vi "Ballistics_PBBA_alpha.vi"() -> ()   [LabVIEW 2012]
doc: "This program is currently beta software. It is designed to address the data requirements defined primarily by the DHB Ballistic Test Report.\n\nThe general operation of this program is based on the Ballistics Version 2005 application developed internally by DuPont as a research tool for the Spruance Plant Ballistics Lab in Richmond, VA.\n\nPlease note that the original trigger control logic was modified and no longer depends on a safety interlock system to enable operation of a ballistic test.\n\nDuPont makes no warranties and assumes no liabilities in connection with any use of this program."
uses:
  <vilib>/Utility/NIReport.llb/NI_report.lvclass
  <vilib>/addons/database/NI_Database_API.lvlib
  <vilib>/addons/database/Connection.llb/Conn Execute.vi
  <vilib>/addons/database/Recordset.llb/Rec Destroy - Connection.vi
  <vilib>/Utility/config.llb/NI_LVConfig.lvlib
  <vilib>/Utility/config.llb/Write Key (I32).vi
  <vilib>/addons/database/Connection.llb/DB Tools Open Connec (String).vi
  <vilib>/Analysis/NI_AALBase.lvlib
  Instance           1 29Saved   Ballistics_PBBA_alpha .vi
  <vilib>/Utility/NIReport.llb/Append Text Table to Report (wrap).vi
  <vilib>/Utility/NIReport.llb/Append Report Text (str wrap).vi
  Shot Record.ctl
panel:
  out "dbConn":string caption="Database Connection"
  in  "RESET":bool
  in  "EXIT":bool
  in  "message control":bool=TRUE
  in  "String":string="Ply Data Not Entered"
  in  "mainTabCntrl":T1(tab)=enum."MEASURE"
  in  "setupTabCntrl":T2(tab)
  in  "weight(gr)":u16(ring) caption="Weight (gr)" items=["2", "4", "16", "17", "44", "64", "124", "158", "240"]
  in  "clayAverage":sgl caption="Clay Average"
  in  "clayCalib":string="##-##-##-##-##" caption="Calibration"
  in  "clayTemp":i16=65 caption="Clay Temperature"
  in  "Room Temperature":i32
  in  "Room Humidity":i32
  in  "Sample ID":string
  in  "Test Conditions":u16(ring) items=["Dry", "Wet", "Hot 160 DEG. F", "Cold", "WEAPON LUBRICANT", "MOTOR OIL", "CONDITIONED", "ACCELERATED AGEING"]
  in  "Panel Dimensions":u16(ring) items=["15x15", "HELMET", "12x15", "16X16", "18X18", "20X16", "15x18", "24x24", "13X13", "7.5x7.5", "VEST PANEL", "12X12", "101/4x113/4", "15X16", "26X26", "NOT APPLICABLE", "8.5x11", "CHEST PLATE"]
  in  "Submitter":u16(ring) items=["other"]
  in  "Test Comments":string
  in  "Panel Backing":u16(ring)=1 items=["miscellaneous", "Clay (ROMA Plastilina # 1)", "Aluminum, 24 ga. (.020,.2024-T3) Witness Plate", "None"]
  in  "Threat 2":u16(ring) caption="Threat" items=["16-grain,  saboted RCC,.308cal.SAAMI test bbl.,DC", "17-grain,sabot.Type 1,FSP,.308cal.SAAMI test bbl.,DC", "17-grain,sabot.Type 2,FSP,.308cal.SAAMI test bbl.,DC", "2-grain, saboted RCC FSP,.223cal.SAAMI test bbl.,DC", "4-grain, saboted RCC FSP ,.223cal.SAAMI test bbl.,DC", "44-grain,sabot.      FSP,.458cal.SAAMI test bbl.,DC", "64-grain,sabot.  RCC,.458cal.SAAMI test bbl.,DC"]
  in  "recorder":u16(ring) caption="Recorder" items=["Mike Slate", "Dan Kraus", "Pat Fitzgerald", "Other"]
  in  "shooter":u16(ring) caption="Shooter" items=["Mike Slate", "Pat Fitzgerald", "Other"]
  in  "rangeNum":u16(ring) caption="Range #" items=["1", "2", "Other"]
  in  "barrelLen":u16(ring) caption="Barrel Length" items=["24", "10", "Other"]
  in  "projectile":u16(ring) caption="Projectile" items=["RCC", ".357mag JSP", ".44mag SJHP", "9mm FMJ", "22cal FSP", "7.62 FMJ"]
  in  "weapon":u16(ring) caption="Weapon" items=["Universal Receiver", "Other"]
  in  "minV50":i32=1500 caption="Minimum V50"
  in  "covering":u16(ring) caption="Ballistic Cover" items=["Other", "RipStop"]
  out "totalBAW":sgl caption="Total BAW" format="%.2f"
  in  "totalSampleWt":sgl caption="Total Weight" format="%.2f"
  in  "modelNum":string caption="Model #"
  in  "serialNum":string caption="Serial #"
  in  "workType":u16(ring) caption="Type of Work" items=["R&D", "QC", "Other"]
  in  "projNum":string caption="Project #"
  in  "projName":string caption="Project Name"
  in  "standard":u16(ring)=1 caption="Standard" items=["NIJ 0101.04", "MIL-STD-662F", "Other"]
  in  "Powder Type":u16(ring) items=["WINCHESTER-231", "Alliant Herc. Bullseye", "Power Pistol", "ACCURATE, NO.9", "ACCURATE, NO. 2", "IMR-4756", "OTHER", "WINCHESTER-296", "Alliant 2400", "IMR-4198", "IMR-4895", "Hi-Skor 700x", "Hi-Skor 800x", "International Clay's", "Winchester Ball", "Hercules"]
  in  "ballistician":u16(ring) caption="Ballistician" items=["n.a."]
  in  "Method":u16(ring) items=["V50", "N.I.J.", "Quasi N.I.J.", "VsVr", "CUSUM", "V(0)", "V(0) @ 1450", "V(0) @ 1500", "V(0) @ 1550"]
  out "fab6_totalWt":sgl caption="Fab6 Wt" min=0 max=99 step=5 format="%.2f"
  out "fab5_totalWt":sgl caption="Fab5 Wt" min=0 max=99 step=5 format="%.2f"
  out "fab4_totalWt":sgl caption="Fab4 Wt" min=0 max=99 step=5 format="%.2f"
  out "fab3_totalWt":sgl caption="Fab3 Wt" min=0 max=99 step=5 format="%.2f"
  out "fab2_totalWt":sgl caption="Fab2 Wt" min=0 max=99 step=5 format="%.2f"
  out "fab1_totalWt":sgl caption="Fab1 Wt" min=0 max=99 step=5 format="%.2f"
  in  "Layers":T3(array[cluster])=[{"Ply Description"=0, "Layer Comments"="", "Number of Plies"=20, "Fabric.vendor"=1, "Fabric.styleNum"=1, "Fabric.fiber"=1, "Fabric.denier"=1, "Fabric.pickWeave"=0, "Fabric.finish"=0, "LotNum"="n/a", "RollNum"="n/a", "ozPerYd2"=20.0, "Fabric.stitch"=0}] {"Fabric.stitch" items=["Corners", "Other", "n/a"]; "ozPerYd2" min=0 max=99 step=5; "Fabric.finish" items=["Greige", "ML", "WRT", "Other"]; "Fabric.pickWeave" items=["18x18 / Plain", "20x20 / Plain", "24x24 / Stn,Pln,Sn", "Other"]; "Fabric.denier" items=["600", "800", "840", "1000", "Other"]; "Fabric.fiber" items=["Kevlar", "Twaron", "Other"]; "Fabric.styleNum" items=["8606", "A087", "8542B", "Other"]; "Fabric.vendor" items=["TTI", "Barrday", "TexTech", "Other"]; "Number of Plies" min=0 max=99 step=5; "Ply Description" items=["ANY STYLE", "none"]}
  in  "Fabric Description":string
  out "Total Number of Layers":i32=1 caption="Total Number\nof Layers" min=0 max=100 step=5
  in  "Panel Technician":u16(ring) items=["Not Known", "none", "POINT BLANK"]
  in  "Weight of Panel":dbl format="%.4f"
  in  "Areal density text":string
  in  "Areal Density":dbl format="%.2f"
  in  "Thickness":dbl format="%.2f"
  in  "Manufacturer":u16(ring) caption="Mfr" items=["Point Blank-Marine Interceptor", "Other"]
  in  "Type":u16(ring) items=["none"]
  in  "Panel Type":u16(ring) items=["FABRIC ARMOR", "COMPOSITE ARMOR", "LG.RIGHT FRONT VEST PANEL", "HELMET", "N.A."]
  in  "Panel Stitch":u16(ring) items=["TEST PANEL/NORMAL STITCH", "TEST PANEL/CUSTOM STITCH", "VEST PANEL/CUSTOM STITCH", "HARD PANEL", "CAR ARMOR LAMINATE PANEL", "N.A."]
  in  "Next Shot":bool
  in  "Delete Button":bool
  in  "SHOTS":T4[](array[typedef]) {"UncorrectedAvgVel_PB" format="%.1f"; "strikeVel_PB" format="%.1f"; "velLoss_PB" format="%.1f"; "avgVel_PB" format="%.1f"; "Redundant_Velocity" format="%.1f"; "Energy Loss (J)" format="%.3e"; "Projectile Mass" min=0 step=1 format="%.4f"; "Corrected residual" format="%.2f"; "Uncorrected Residual" format="%.2f"; "Corrected Impact" format="%.2f"; "Uncorrected Impact" format="%.2f"; "Shot Angle" max=90 step=1; "SHOT STATUS" items=["Partial", "Complete"]; "IMPACT VELOCITY" min=0 max=10000 step=0.1 format="%.1f"; "Barrel Temperature" format="%.1f"; "Powder Loading" format="%.4f"; "RESIDUAL  VELOCITY" min=0 max=10000 step=0.1 format="%.1f"}
  in  "reread":bool
  out "Shot":i32
  out "Panel":i32
  out "rangeOfResults":i32 caption="Range of Results" min=0 max=10000 step=1
  out "lowComplete":i32 caption="LOW Complete" min=0 max=10000 step=1
  out "highPartial":i32 caption="HIGH Partial" min=0 max=10000 step=1
  out "Avg/speed":sgl caption="Average" min=0 max=10000 step=0.1 format="%.1f"
  in  "Current/avg/speed":sgl caption="REDUNDANT VELOCITY" min=0 max=1000000 step=0.1 format="%.1f"
  out "Redundant/speed":sgl caption="Chronograph 2" min=0 max=10000 step=0.1 format="%.1f"
  in  "backfacedia":sgl
  in  "backdepth":sgl
  out "% Difference":sgl=0.991641 format="%.1f"
  out "zmr 2":sgl caption="Z.M.R." format="%.1f"
  out "Pairs":i16 min=0 max=100 step=1
  out "computed_V50":sgl caption="Value" format="%.1f"
  in  "MaxDeviation":sgl=125.0 caption="Maximum\nDeviation" min=0 max=200 step=25 format="%.1f"
  in  "B.F.S (mm)":u16 caption="B.F.S"
  in  "N.I.J":u16(ring) items=["Not Tested", "PASS", "FAIL"]
  in  "Projectile Mass":sgl=7.12788 caption="Projectile Mass\n(grams)" min=0 step=1 format="%.4f"
  in  "Shot Angle":u16 max=90 step=1
  in  "Powder Loading":sgl min=0 max=100 step=0.1 format="%.3f"
  in  "Shot Decription":string
  in  "Barrel Temp":sgl format="%.1f"
  out "Residual factor":sgl=1.0 caption="Residual" min=0 max=1 format="%.5f"
  out "Impact factor":sgl=1.0 caption="Impact" min=0 max=1 format="%.5f"
  out "DC_ factor":sgl=1.0 caption="Midpoint of\nChrono 1 and 2" format="%.4f"
  in  "Drag Corrected":bool=TRUE
  in  "Current/redundant/speed":sgl caption="REDUNDANT VELOCITY" min=0 max=1000000 step=0.1 format="%.1f"
  out "currentDateTime":string
  in  "Current/residual/speed":sgl min=0 max=10000 step=0.1 format="%.1f"
  in  "Current/sthotstatus":u16(ring) items=["Partial", "Complete"]
  in  "Current/impact/speed":sgl min=0 max=10000 step=0.1 format="%.1f"
  out "BACKFACE DEPTH":sgl caption="Backface\nDepth" min=0 max=200 step=5
  out "BACKFACE DIAMETER":sgl caption="Backface\nDiameter" min=0 max=100 step=5
  in  "Reject shot":bool
  in  "Accept Data":bool
  out "SUBMIT DATE/TIME":string
  out "residual/speed":sgl caption="Residual" min=0 max=10000 step=0.1 format="%.1f"
  out "SHOT STATUS":u16(ring) caption="Penetration" items=["Partial", "Complete"]
  out "Impact/speed":sgl caption="Chronograph 1" min=0 max=10000 step=0.1 format="%.1f"
  in  "Table of Shots":string[][](table) caption="Shot Table"
  in  "RANGE RESET":bool
  in  "Save":bool
  out "Data retrieval":string="\nWORKING"
  out "ActualNumRecs":i32=1001 caption="Actual Number of \nRecords Returned"
  in  "latest Date":string="1/1/2100"
  in  "DATE 3":string="1/1/2100"
  in  "DATE 2":string="1/1/1900"
  in  "velocity-loading":bool
  in  "Panel Search":bool
  in  "Earliest Date":string="1/1/1900"
  in  "maxRecs":u16=1001 min=1 max=10000 step=100
  out "v50 data 2":string[][](table)
  out "In Control":bool=TRUE caption="Control Status"
  in  "queryThreat":u16(ring) caption="Threat" items=["115-GRAIN,9mm LUGER,REFERENCE ROUND,10\" .38 cal TEST BBL.", "158-grain,WIN. 357 MAG, JHP REFERENCE ROUND, 10\" SAMMI TEST BBL.", "180-grain,WIN. 308 POWER-POINT REFERENCE ROUND, 308 TEST BBL.", "240-grain,REM. .44 mag, JSP REFERENCE ROUND, 8\" SAMMI TEST BBL."]
  in  "Powder":string="bul"
  out "St. Deviation":dbl=31.606020957071 format="%.1f"
  out "Latest Velocity":dbl=1314.9 format="%.1f"
  out "Average Velocity":dbl=1297.749514563107 format="%.1f"
  out "Previous V50 Data":cluster{dbl, dbl, dbl[][]}(graph)={0.0, 1.0, []}
  in  "Threat":string
  out "Velocity versus Loading":cluster{dbl[], dbl[]}(graph)
  out "v50 data":string[][](table)
  in  "Residual  Timer":i16=2 min=0 max=3 step=1
  in  "Redundant Timer":i16=1 min=0 max=3 step=1
  in  "Impact Timer":i16 min=0 max=3 step=1
  in  "DAQ Card":i16=1
  out "Device S/N":string caption="Timing Device S/N"
  in  "switch":bool
  in  "Stop Program":bool
  in  "old drag":bool
  out "Partial":sgl[](array[numeric]) format="%.2f"
  out "factor array":sgl[](array[numeric]) format="%.4f"
  out "Complete":sgl[](array[numeric]) format="%.2f"
  in  "Contact Shot Report":bool
  in  "Old_Shots":T4[](array[typedef]) {"UncorrectedAvgVel_PB" format="%.1f"; "strikeVel_PB" format="%.1f"; "velLoss_PB" format="%.1f"; "avgVel_PB" format="%.1f"; "Redundant_Velocity" format="%.1f"; "Energy Loss (J)" format="%.3e"; "Projectile Mass" min=0 step=1 format="%.4f"; "Corrected residual" format="%.2f"; "Uncorrected Residual" format="%.2f"; "Corrected Impact" format="%.2f"; "Uncorrected Impact" format="%.2f"; "Shot Angle" max=90 step=1; "SHOT STATUS" items=["Partial", "Complete"]; "IMPACT VELOCITY" min=0 max=10000 step=0.1 format="%.1f"; "Barrel Temperature" format="%.1f"; "Powder Loading" format="%.4f"; "RESIDUAL  VELOCITY" min=0 max=10000 step=0.1 format="%.1f"}
  in  "old threat":u16
  out "Z.M.R.":sgl min=0 step=0.1 format="%.1f"
  in  "Residual/Target Dist":sgl=7.083333 format="%.2f"
  out "Residual/Separation":sgl=4.0 format="%.2f"
  in  "Impac/Target Dist":sgl=7.083333 format="%.2f"
  out "Barrel to Screen Distance":sgl=7.8333 format="%.2f"
  out "Impact/Separation":sgl=4.0 format="%.2f"
  out "plytypes":u16=1
  out "Corrected Impact":sgl=44.292404 format="%.2f"
  out "Corrected Residual":sgl format="%.2f"
  out "correction coefficient":sgl format="%.8f"
  out "Red/ID":u32=84017153 format="%.0x"
  out "residual/ID":u32=83951617 format="%.0x"
  out "impact/ID":u32=83886081 format="%.0x"
  in  "Version":dbl format="%.2f"
  in  "percent warning":sgl=1.0 format="%.2f"
  out "number of partials":i32=2
  out "number of completes":i32=3
  out "conversion factor":sgl=0.3048037 format="%.5f"
  in  "mid_to_targ_dist":sgl caption="Midpoint To Target Distance"
  out "Corrected Redundant":sgl=44.292404 format="%.2f"
  out "Corrected Average":sgl=44.292404 format="%.2f"
  out "Shot Graph":cluster{i32[], sgl[]}[](graph)
  in  "Data Source":u16(ring)=2 items=["Simulated", "Radar", "Screens"]
  out "Distance Units":string
  out "Weight Units":string
  in  "Report_PB":bool caption="Report"
  in  "Add Disclaimer":bool
  in  "Report":bool
  in  "Report Path":path=path "c:/ballistics"
  # "The bottom section of this pane contains new fields\nspecified by the PBBA Test reports.\n\nSome of the fields from the DuPont grouping (as marked \nin the top section) are also needed to complete a report."
  # "GENERAL"
  # "SAMPLE"
  # "THREAT"
  # "RANGE"
  # "lbs."
  # "° F"
  # "lbs."
  # "mm"
  # "mm"
  # "Strike Face -------------------------------------------------------- Model Construction --------------------------------------------------------> Body Side"
  # "[----- Fabric #1 -------------- Fabric #2 -------------- Fabric #3 -------------- Fabric #4 -------------- Fabric #5 -------------- Fabric #6 -----]"
  # "Ply Description"
  # "Layer Comments"
  # "# of Plies"
  # "Vendor"
  # "Style #"
  # "Fiber"
  # "Denier"
  # "Pick / Weave"
  # "Finish"
  # "Lot#"
  # "Roll#"
  # "oz/yd²"
  # "Stitch"
  # "Total Weight"
  # "Edit any non-date field by placing cursor in field. \n\nProperties not listed are controlled by the current shot, test description or Fabric information.  \nIf the entry is changed for the current shot, then all previous shots are changed"
  # "Current Shot Data"
  # "(mm)"
  # "V50"
  # "NOTE: Number of  plies must be entered in FABRIC INFORMATION to enable saving"
  # "Point Blank Body Armor Ballistics Test Station"
  # "Last Assigned\nRecord Numbers"
  # "Correction Factors"
  # "CUSUM HISTORY"
  # "SHOT DATA"
  # "Max Records Returned\n (up to 10,000)"
  # "Date Range"
  # "(Form: 1/25/2000)"
  # "Date Range"
  # "Begin date"
  # "End Date"
  # "(Form: 1/25/2000)"
  # "End Date"
  # "Begin Date"
  # "yes"
  # "No"
  # "PBBA"
  # "Point Blank Body Armor\nBallistics Test Station\n\nVersion 1.00 ALPHA\n\nOctober 2006"
  # "To arrange for technical support, contact\n\nPat Fitzgerald or Mark Hartsky\n\nDuPont Company"
  # "This program is currently beta software. It is designed to address the data requirements defined primarily by the DHB Ballistic Test Report.\n\nThe general operation of this program is based on the Ballistics Version 2005 application developed internally by DuPont as a research tool for the Spruance Plant Ballistics Lab in Richmond, VA.\n\nPlease note that the original trigger control logic was modified and no longer depends on a safety interlock system to enable operation of a ballistic test.\n\nDuPont makes no warranties and assumes no liabilities in connection with any use of this program."
  # "Yes"
  # "No"
  # "DuPont"
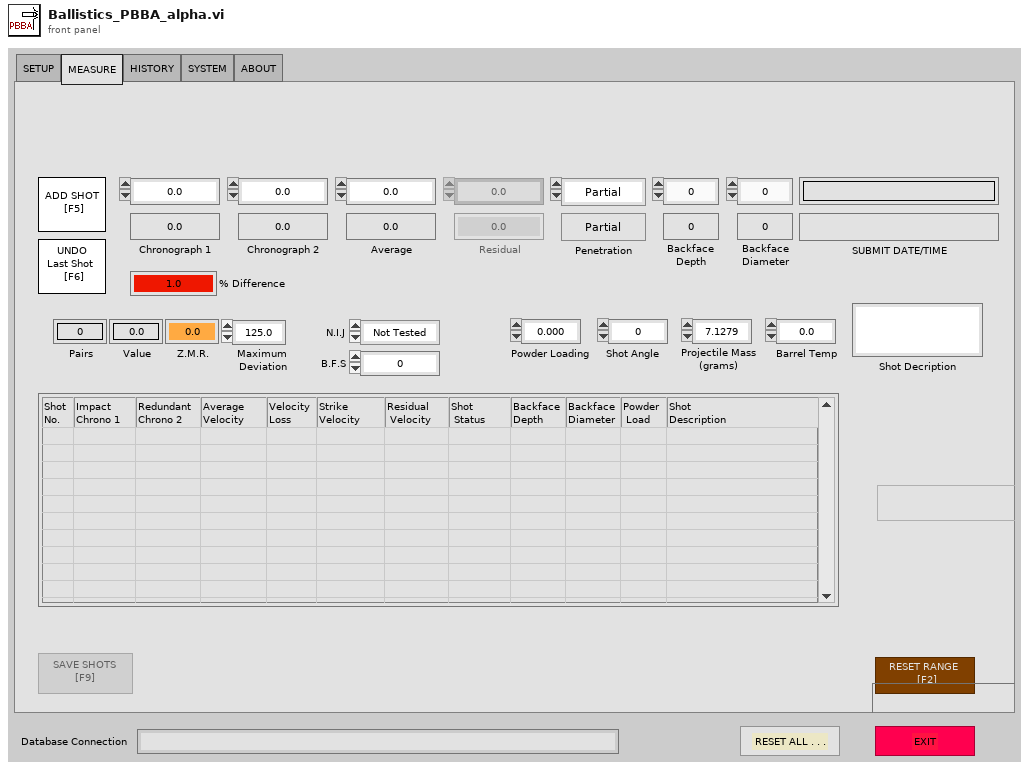
[diagram p1: front panel]
types:
  T1 = enum32{"SETUP", "MEASURE", "HISTORY", "SYSTEM", "ABOUT"}
  T2 = enum32{"Test Description", "Fabric Information", "Edit Previous Shots"}
  T3 = cluster{"Ply Description":u16, "Layer Comments":string, "Number of Plies":i32, "Fabric.vendor":u16, "Fabric.styleNum":u16, "Fabric.fiber":u16, "Fabric.denier":u16, "Fabric.pickWeave":u16, "Fabric.finish":u16, "LotNum":string, "RollNum":string, "ozPerYd2":sgl, "Fabric.stitch":u16}[]
  T4 = typedef "Shot Record.ctl" = cluster{"avgVel_PB":sgl, "IMPACT VELOCITY":sgl, "RESIDUAL  VELOCITY ":sgl, "Shot Description":string, "Powder Loading ":sgl, "Barrel Temperature":sgl, "TIME / DATE":string, "shot order":i32, "SHOT STATUS":u16, "Shot Angle":u16, "Uncorrected Impact":sgl, "Corrected Impact":sgl, "Uncorrected Residual":sgl, "Corrected residual":sgl, "Projectile Mass":sgl, "usedv50":bool, "Energy Loss (J)":sgl, "BackFace\nDepth":sgl, "BackFace\nDiameter":sgl, "Redundant_Velocity":sgl, "velLoss_PB":sgl, "strikeVel_PB":sgl, "UncorrectedRed_PB":sgl, "CorrectedRed_PB":sgl, "UncorrectedAvgVel_PB":sgl}
  T5 = cluster{"impactCntrID":u32, "redundantCntrID":u32, "residualCntrID":u32}
  T6 = cluster{"Charset (-1)":i16, "Weight (-1)":i16, "Name":string, "Size":string}
  T7 = cluster{"Italic":enum16{"Italic Unchanged", "Italic On", "Italic Off"}, "Strike Through":enum16{"Strike Through Unchanged", "Strike Through On", "Strike Through Off"}, "Underline":enum16{"Underline Unchanged", "Underline On", "Underline Off"}, "Bold":enum16{"Bold Unchanged", "Bold On", "Bold Off"}}
  T8 = enum16{"Standard Report", "HTML", "Word", "Excel"}
  T9 = typedef "NI_Database_API.lvlib/Conn ObjectReference.ctl" = refnum<k1>
  T10 = typedef "NI_Database_API.lvlib/Rec ObjectReference.ctl" = refnum<k1>
  T11 = typedef "NI_LVConfig.lvlib/Config Data RefNum.ctl" = refnum<k1>
  T12 = cluster{"task ID out":u32, "task ID out":u32, "task ID out":u32}
  T13 = cluster{"Sample ID":string, "element":string, "element":string, "serialNum":string, "modelNum":string, string, string, string, "element":string, string}
  T14 = cluster{string, string, string, "clayCalib":string, string}
  T15 = cluster{"element":string, "element":string, "element":string, "element":string, "element":string, string, "element":string, "element":string, "element":string}
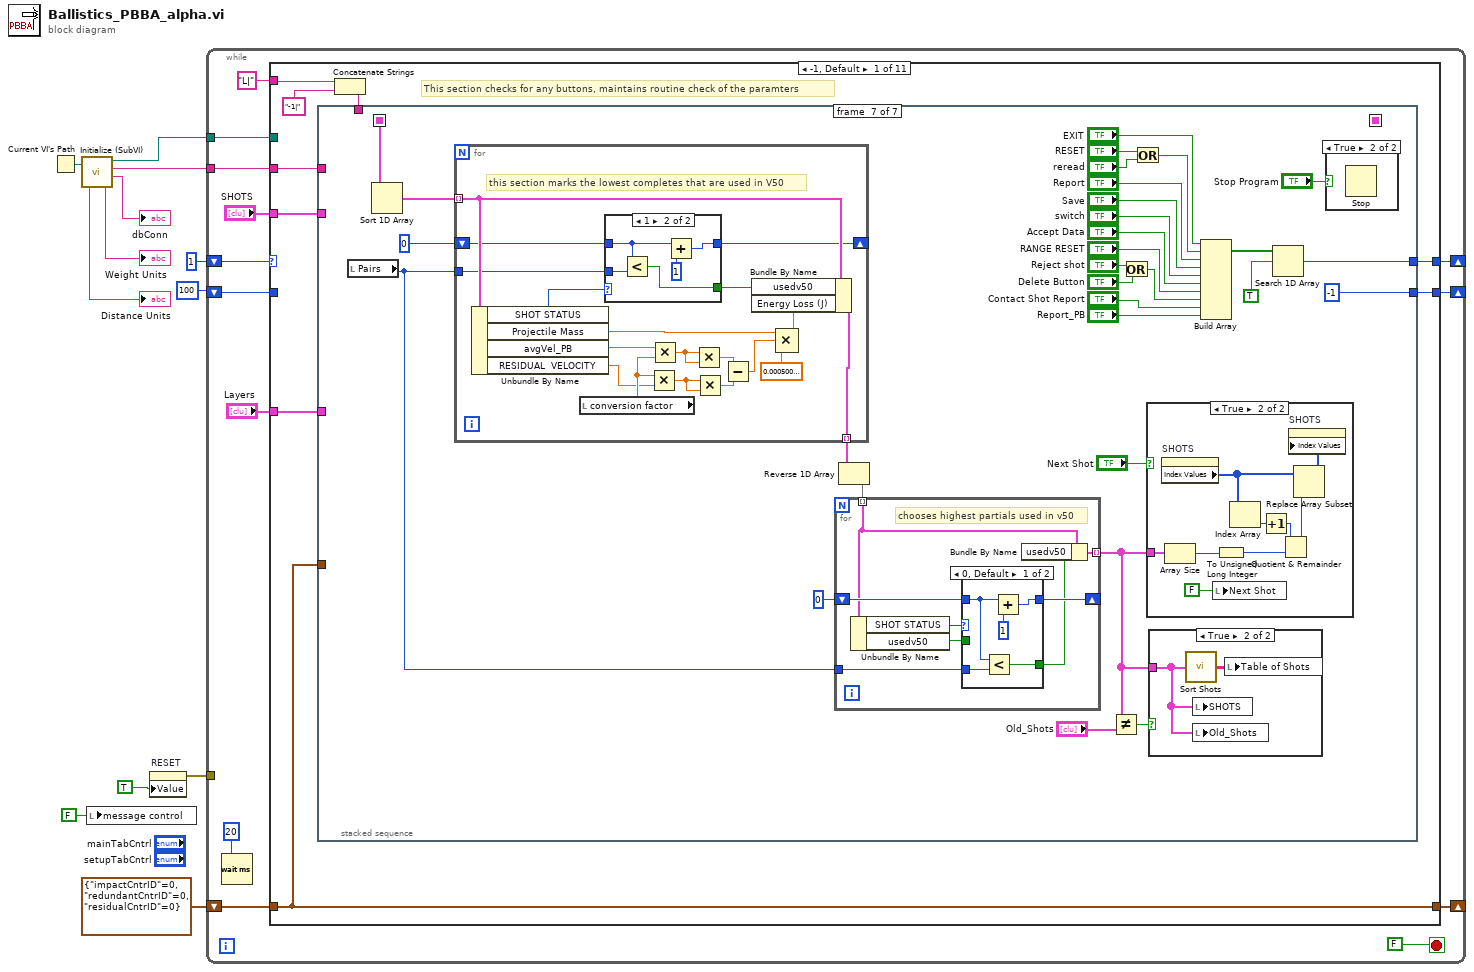
[diagram p0: block diagram]
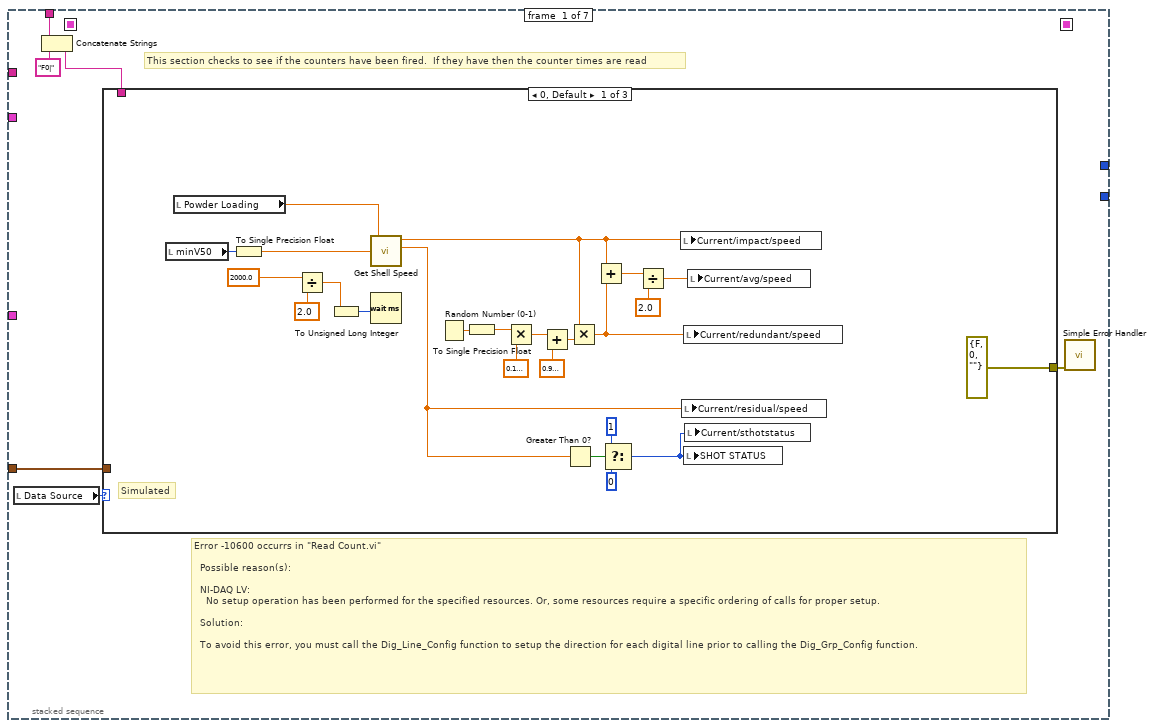
[diagram p2: hidden frame]
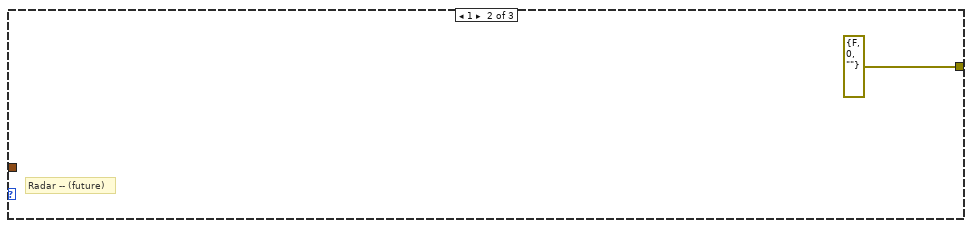
[diagram p3: hidden frame]
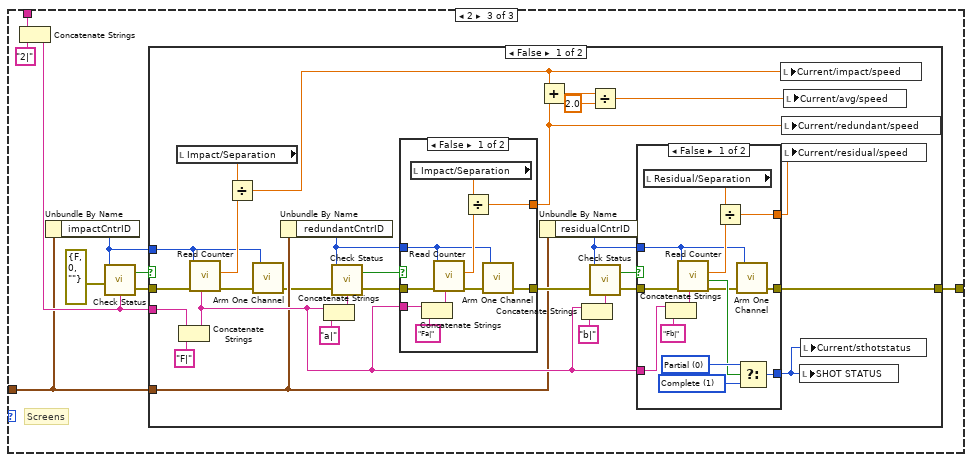
[diagram p4: hidden frame]
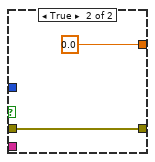
[diagram p5: hidden frame]
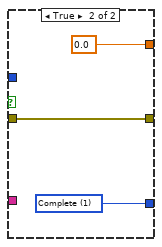
[diagram p6: hidden frame]
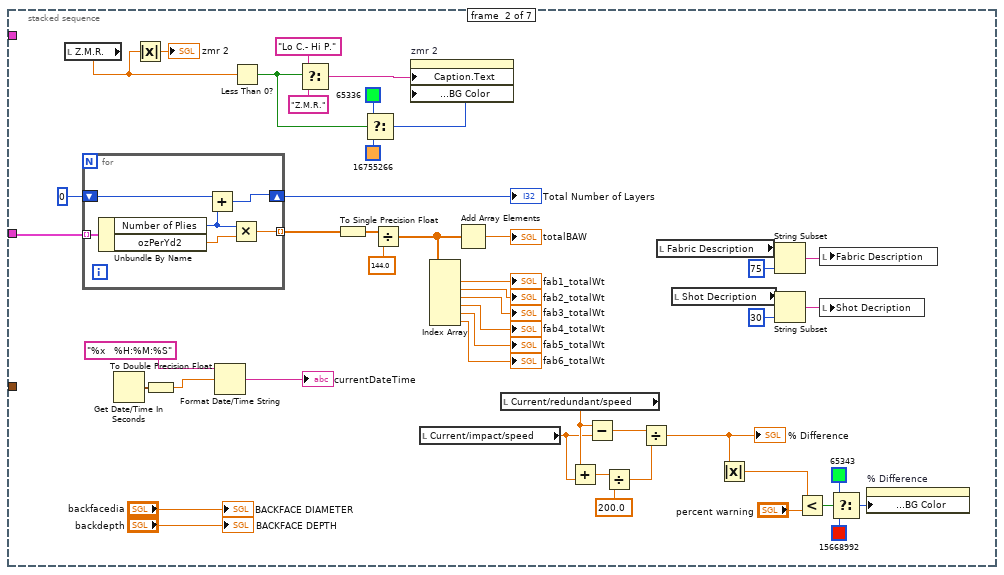
[diagram p8: hidden frame]
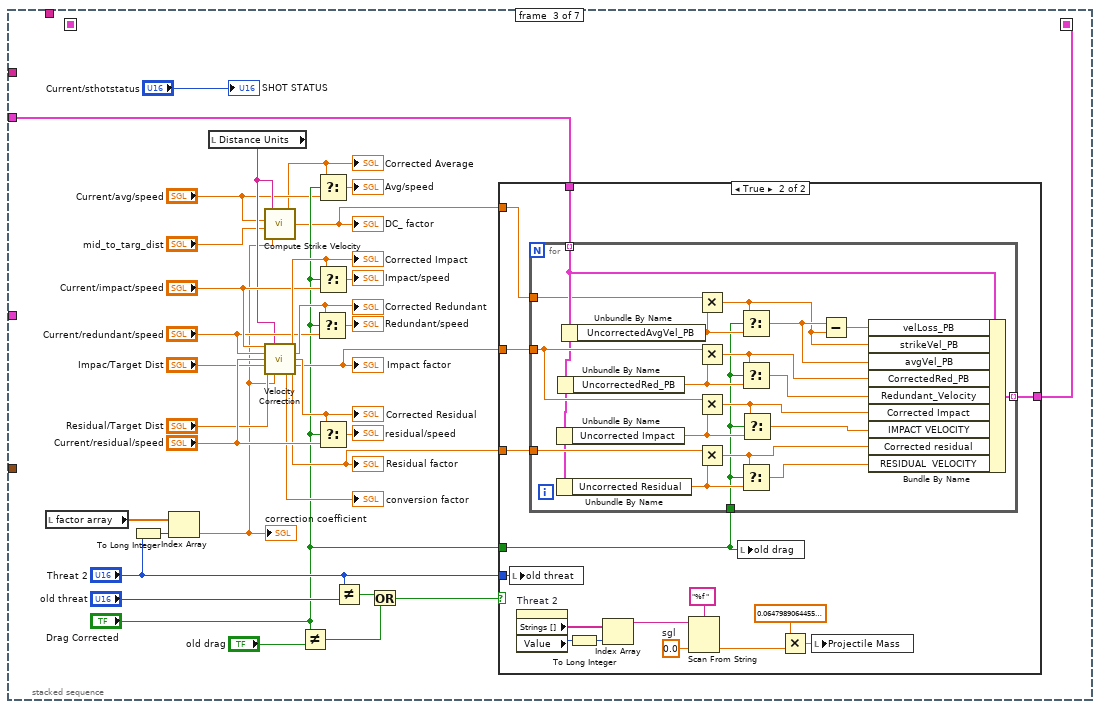
[diagram p9: hidden frame]
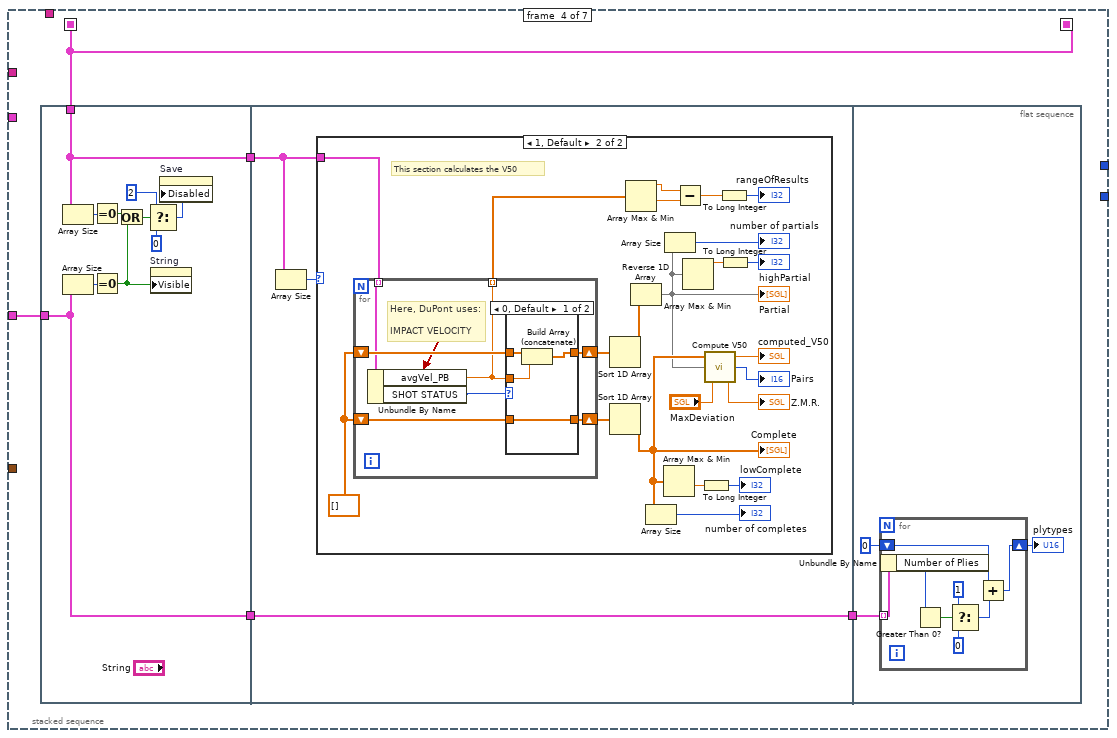
[diagram p11: hidden frame]
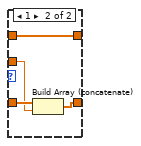
[diagram p13: hidden frame]
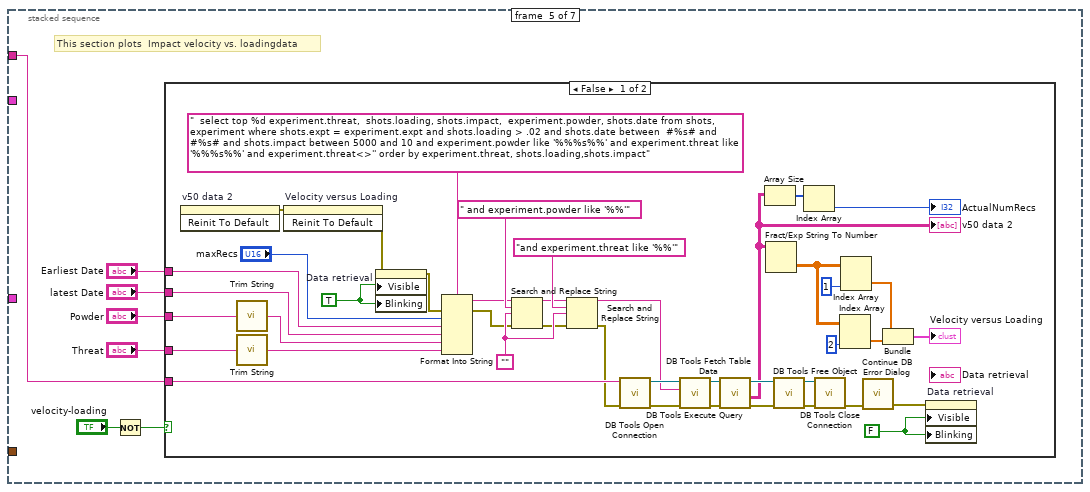
[diagram p14: hidden frame]
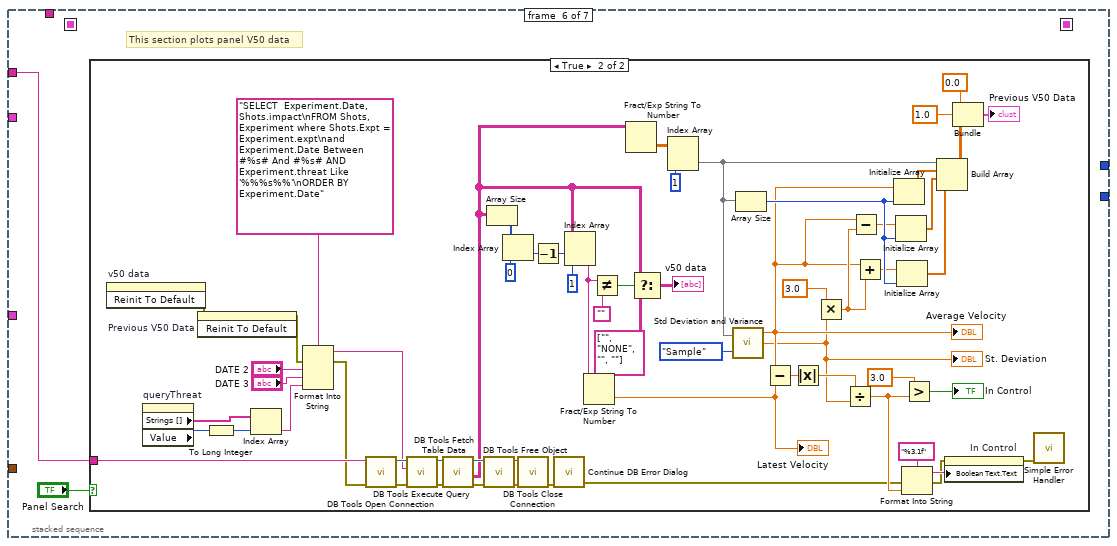
[diagram p16: hidden frame]
diagram:
  n1 = Current VI's Path() -> (path=w1:path)
  n2 = call "Initialize (SubVI).vi"("appended path IN"=w1) -> ("Distance Units"=→"Distance Units":string, "appended path OUT"=w6:path, "connectString"=w9:string, "Database Connection"=→"dbConn":string, "Weight Units"=→"Weight Units":string)
  n3 = local write "message control"(FALSE) -> ()
  n4 = property on="RESET" class="Bool (strict)"("Value"=TRUE ("RESET")) -> (error out=w7:errorcluster)  [unwired: 2 in, 1 out]
  n5 = while {
    shift-left: 100 -> [w21]
    shift-right: [w22] -> _
    shift-left: 1 ("index of element") -> [w25]
    shift-right: [w23] -> _
    tunnel: w6 -> [w18]
    tunnel: w9 -> [w17]
    tunnel: w7 -> [_]
    shift-right: [w15] -> _
    shift-left: T5 {"impactCntrID"=0, "redundantCntrID"=0, "residualCntrID"=0} -> [w14]
    stop <- FALSE stop-if-true
    n6 = Wait (ms)(milliseconds to wait=u32 20 ("millisecond timer value")) -> ()  [unwired: 1 out]
    n7 = case shown="-1, Default" w25 {
      tunnel: [w32 w517 w522 w751 w774 w1032 w1074 w1082 w1126 w1244 w1289] -> w23
      tunnel: [w33 w517 w522 w751 w773 w1032 w1074 w1082 w1126 w1244 w1289] -> w22
      tunnel: w21 -> [_ _ w525 _ _ _ _ _ _ _ _]
      tunnel: "SHOTS" -> [w34 _ _ _ w772 w1022 w1061 _ w1124 _ w1281]
      tunnel: w18 -> [_ _ w524 _ w766 _ _ _ _ _ _]
      tunnel: w17 -> [w31 _ w523 _ w770 _ _ _ _ _ _]
      tunnel: "L|" -> [w30 _ _ _ _ _ _ w1078 _ _ _]
      tunnel: [w27 w516 w521 w629 w769 w1020 w1048 w1077 w1121 w1175 w1288] -> w15
      tunnel: w14 -> [w27 w516 w521 w629 w769 w1020 w1048 w1076 w1121 w1175 w1288]
      tunnel: "Layers" -> [w26 _ _ _ w768 _ _ _ _ _ w1282]
      frame -1, Default {
        # "This section checks for any buttons, maintains routine check of the paramters"
        n8 = Concatenate Strings(w30, "-1|") -> (w28:string)
        n9 = stacked-sequence {
          seq-local: [_ _ _ w261 _ _ _] -> [_ _ _ _ _ _ w446]
          seq-local: [_ _ w211 _ _ _ _] -> [_ _ _ w261 _ _ _]
          tunnel: w34 -> [_ _ w198 _ _ _ _]
          tunnel: [_ _ _ _ _ _ w450] -> w32
          tunnel: [_ _ _ _ _ _ -1] -> w33
          tunnel: w31 -> [_ _ _ _ w323 w373 _]
          tunnel: w28 -> [w38 _ _ _ _ _ _]
          tunnel: w27 -> [w35 _ _ _ _ _ _]
          tunnel: w26 -> [_ w134 _ w259 _ _ _]
          frame #0 {
            # "Error -10600 occurrs in \"Read Count.vi\"\n\n  Possible reason(s):\n\n  NI-DAQ LV:\n    No setup operation has been performed for the specified resources. Or, some resources require a specific ordering of calls for proper setup.  \n\n  Solution: \n\n  To avoid this error, you must call the Dig_Line_Config function to setup the direction for each digital line prior to calling the Dig_Grp_Config function."
            # "This section checks to see if the counters have been fired.  If they have then the counter times are read"
            n10 = local read "Data Source"() -> (w40:u16)
            n11 = Concatenate Strings(w38, "F0|") -> (w36:string)
            n12 = case shown="0, Default" w40 {
              tunnel: [errorcluster {"status"=FALSE, "code"=0, "source"=""} ("error out") errorcluster {"status"=FALSE, "code"=0, "source"=""} ("error out") w74] -> w39
              tunnel: w36 -> [_ _ w70]
              tunnel: w35 -> [_ _ w66]
              frame 0, Default {
                # "Simulated"
                n13 = local read "minV50"() -> (w43:i32)
                n14 = local read "Powder Loading"() -> (w63:sgl)
                n15 = To Single Precision Float(number=w43) -> (single precision float=w42:sgl)
                n16 = Divide(x=sgl 2000.0, y=sgl 2.0 ("v50")) -> (x/y=w64:sgl)
                n17 = To Unsigned Long Integer(number=w64) -> (unsigned 32bit integer=w50:u32)
                n18 = call "Get Shell Speed.vi"("loading"=w63, "v50"=w42) -> ("impact"=w48:sgl, "residual"=w57:sgl)  [unwired: 2 in, 1 out]
                n19 = Wait (ms)(milliseconds to wait=w50) -> ()  [unwired: 1 out]
                n20 = Random Number (0-1)() -> (number: 0 to 1=w55:dbl)
                n21 = To Single Precision Float(number=w55) -> (single precision float=w49:sgl)
                n22 = Multiply(x=w49, y=sgl 0.1) -> (x*y=w54:sgl)
                n23 = Add(x=w54, y=sgl 0.95) -> (x+y=w52:sgl)
                n24 = Greater Than 0?(x=w57) -> (x > 0?=w60:bool)
                n25 = Multiply(x=w48, y=w52) -> (x*y=w47:sgl)
                n26 = Add(x=w48, y=w47) -> (x+y=w45:sgl)
                n27 = Select(t=u16 1, s=w60, f=u16 0) -> (s? t:f=w58:u16)
                n28 = Divide(x=w45, y=sgl 2.0 ("v50")) -> (x/y=w44:sgl)
                n29 = local write "Current/impact/speed"(w48) -> ()
                n30 = local write "Current/residual/speed"(w57) -> ()
                n31 = local write "Current/redundant/speed"(w47) -> ()
                n32 = local write "SHOT STATUS"(w58) -> ()
                n33 = local write "Current/sthotstatus"(w58) -> ()
                n34 = local write "Current/avg/speed"(w44) -> ()
              }
              frame 1 {
                # "Radar -- (future)"
              }
              frame 2 {
                # "Screens"
                n35 = Concatenate Strings(w70, "2|") -> (w69:string)
                n36 = Unbundle By Name(w66) -> ("impactCntrID"=w67:u32)
                n37 = call "Check Status.vi"("error in (no error)"=errorcluster {"status"=FALSE, "code"=0, "source"=""}, "TL Calling Location"=w69, "Task ID"=w67) -> ("error out"=w72:errorcluster, "Armed?"=w68:bool)  [unwired: 1 in]
                n38 = case shown="False" w68 {
                  tunnel: w72 -> [w97 w133]
                  tunnel: [w98 w133] -> w74
                  tunnel: w67 -> [w80 _]
                  tunnel: w69 -> [w93 _]
                  tunnel: w66 -> [w83 _]
                  frame False {
                    n39 = local read "Impact/Separation"() -> (w101:sgl)
                    n40 = Concatenate Strings(w93, "F|") -> (w88:string)
                    n41 = call "Read Counter.vi"("TL Calling Location"=w88, "error In"=w97, "TASK ID"=w80) -> ("error out"=w82:errorcluster, "time (secs)"=w103:sgl)  [unwired: 3 in, 2 out]
                    n42 = Divide(x=w101, y=w103) -> (x/y=w76:sgl)
                    n43 = call "Arm One Channel.vi"("error IN"=w82, "task ID IN"=w80) -> ("error out"=w81:errorcluster)  [unwired: 2 in, 1 out]
                    n44 = Unbundle By Name(w83) -> ("redundantCntrID"=w85:u32)
                    n45 = Concatenate Strings(w88, "a|") -> (w91:string)
                    n46 = call "Check Status.vi"("error in (no error)"=w81, "TL Calling Location"=w91, "Task ID"=w85) -> ("error out"=w96:errorcluster, "Armed?"=w87:bool)  [unwired: 1 in]
                    n47 = case shown="False" w87 {
                      tunnel: [w111 sgl 0.0] -> w77
                      tunnel: w96 -> [w110 w115]
                      tunnel: [w105 w115] -> w99
                      tunnel: w85 -> [w104 _]
                      tunnel: w88 -> [w108 _]
                      frame False {
                        n48 = local read "Impact/Separation"() -> (w112:sgl)
                        n49 = Concatenate Strings(w108, "Fa|") -> (w107:string)
                        n50 = call "Read Counter.vi"("TL Calling Location"=w107, "error In"=w110, "TASK ID"=w104) -> ("error out"=w106:errorcluster, "time (secs)"=w113:sgl)  [unwired: 3 in, 2 out]
                        n51 = Divide(x=w112, y=w113) -> (x/y=w111:sgl)
                        n52 = call "Arm One Channel.vi"("error IN"=w106, "task ID IN"=w104) -> ("error out"=w105:errorcluster)  [unwired: 2 in, 1 out]
                      }
                      frame True {
                      }
                    }
                    n53 = Add(x=w76, y=w77) -> (x+y=w78:sgl)
                    n54 = Unbundle By Name(w83) -> ("residualCntrID"=w84:u32)
                    n55 = Concatenate Strings(w88, "b|") -> (w89:string)
                    n56 = Divide(x=w78, y=sgl 2.0) -> (x/y=w75:sgl)
                    n57 = call "Check Status.vi"("error in (no error)"=w99, "TL Calling Location"=w89, "Task ID"=w84) -> ("error out"=w95:errorcluster, "Armed?"=w86:bool)  [unwired: 1 in]
                    n58 = case shown="False" w86 {
                      tunnel: w95 -> [w122 w131]
                      tunnel: [w127 w132] -> w102
                      tunnel: w84 -> [w117 _]
                      tunnel: [w116 w131] -> w98
                      tunnel: [w124 sgl 0.0] -> w100
                      tunnel: w88 -> [w119 _]
                      frame False {
                        w128 = u16 1 items=["Partial", "Complete"] ("SHOT STATUS")
                        w129 = u16 0 items=["Partial", "Complete"] ("SHOT STATUS")
                        n59 = local read "Residual/Separation"() -> (w123:sgl)
                        n60 = Concatenate Strings(w119, "Fb|") -> (w120:string)
                        n61 = call "Read Counter.vi"("TL Calling Location"=w120, "error In"=w122, "TASK ID"=w117) -> ("error out"=w118:errorcluster, "counter overflow?"=w125:bool, "time (secs)"=w126:sgl)  [unwired: 3 in, 1 out]
                        n62 = Divide(x=w123, y=w126) -> (x/y=w124:sgl)
                        n63 = call "Arm One Channel.vi"("error IN"=w118, "task ID IN"=w117) -> ("error out"=w116:errorcluster)  [unwired: 2 in, 1 out]
                        n64 = Select(t=w129, s=w125, f=w128) -> (s? t:f=w127:u16)
                      }
                      frame True {
                        w132 = u16 1 items=["Partial", "Complete"] ("SHOT STATUS")
                      }
                    }
                    n65 = local write "Current/impact/speed"(w76) -> ()
                    n66 = local write "Current/redundant/speed"(w77) -> ()
                    n67 = local write "Current/residual/speed"(w100) -> ()
                    n68 = local write "Current/avg/speed"(w75) -> ()
                    n69 = local write "SHOT STATUS"(w102) -> ()
                    n70 = local write "Current/sthotstatus"(w102) -> ()
                  }
                  frame True {
                  }
                }
              }
            }
            n71 = call <vilib>:"Simple Error Handler.vi"("error in (no error)"=w39) -> ()  [unwired: 4 in, 5 out]
          }
          frame #1 {
            n72 = local read "Z.M.R."() -> (w168:sgl)
            n73 = for {
              tunnel: w134 -> [w185] mode=indexing
              shift-right: [w187] -> w179
              shift-left: 0 -> [w186]
              tunnel: [w184] -> w138 mode=indexing
              n74 = Unbundle By Name(w185) -> ("Number of Plies"=w183:i32, "ozPerYd2"=w182:sgl)
              n75 = Add(x=w186, y=w183) -> (x+y=w187:i32)
              n76 = Multiply(x=w183, y=w182) -> (x*y=w184:sgl)
            }
            "Total Number of Layers" <- w179
            n77 = Get Date/Time In Seconds() -> (seconds since 1Jan1904=w146:timestamp)
            n78 = Absolute Value(x=w168) -> (abs(x)=→"zmr 2":sgl)
            n79 = To Double Precision Float(number=w146) -> (double precision float=w176:dbl)
            n80 = Format Date/Time String(time format string (%c)="%x   %H:%M:%S", seconds (now)=w176) -> (date/time string=→"currentDateTime":string)  [unwired: 1 in]
            n81 = Less Than 0?(x=w168) -> (x < 0?=w174:bool)
            n82 = Select(t="Lo C.- Hi P.", s=w174, f="Z.M.R.") -> (s? t:f=w171:string)
            n83 = To Single Precision Float(number=w138) -> (single precision float=w137:sgl[])
            n84 = Select(t=u32 65336, s=w174, f=u32 16755266) -> (s? t:f=w170:u32)
            n85 = Divide(x=w137, y=sgl 144.0) -> (x/y=w136:sgl[])
            n86 = property on="zmr 2" class="DigNum (strict)"("Caption.Text"=w171, "Numeric Text.Text Colors:BG Color"=w170) -> ()  [unwired: 2 in, 2 out]
            n87 = local read "Current/impact/speed"() -> (w165:sgl)
            n88 = Index Array(array=w136) -> (element #1=→"fab1_totalWt":sgl, element #2=→"fab2_totalWt":sgl, element #3=→"fab3_totalWt":sgl, element #4=→"fab4_totalWt":sgl, element #5=→"fab5_totalWt":sgl, element #6=→"fab6_totalWt":sgl)  [unwired: 6 in]
            n89 = Add Array Elements(numeric array=w136) -> (sum=→"totalBAW":sgl)
            n90 = local read "Current/redundant/speed"() -> (w166:sgl)
            n91 = Add(x=w166, y=w165) -> (x+y=w164:sgl)
            n92 = Subtract(x=w166, y=w165) -> (x-y=w167:sgl)
            n93 = Divide(x=w164, y=sgl 200.0) -> (x/y=w163:sgl)
            n94 = Divide(x=w167, y=w163) -> (x/y=w159:sgl)
            "% Difference" <- w159
            n95 = local read "Fabric Description"() -> (w152:string)
            n96 = local read "Shot Decription"() -> (w149:string)
            n97 = Absolute Value(x=w159) -> (abs(x)=w156:sgl)
            n98 = String Subset(string=w152, length (rest)=75 ("length (rest)")) -> (substring=w151:string)  [unwired: 1 in]
            n99 = String Subset(string=w149, length (rest)=30 ("length (rest)")) -> (substring=w147:string)  [unwired: 1 in]
            n100 = Less?(x=w156, y="percent warning") -> (x < y?=w157:bool)
            n101 = local write "Fabric Description"(w151) -> ()
            n102 = local write "Shot Decription"(w147) -> ()
            n103 = Select(t=u32 65343, s=w157, f=u32 15668992) -> (s? t:f=w155:u32)
            n104 = property on="% Difference" class="DigNum (strict)"("Numeric Text.Text Colors:BG Color"=w155) -> ()  [unwired: 2 in, 2 out]
            "BACKFACE DIAMETER" <- "backfacedia"
            "BACKFACE DEPTH" <- "backdepth"
          }
          frame #2 {
            n105 = local read "factor array"() -> (w219:sgl[])
            n106 = To Long Integer(number="Threat 2") -> (32bit integer=w203:i32)
            n107 = Index Array(array=w219, index=w203) -> (element=w193:sgl)
            "correction coefficient" <- w193
            n108 = local read "Distance Units"() -> (w195:string)
            n109 = call "Compute Strike Velocity.vi"("drag coefficient"=w193, "decay distance"="mid_to_targ_dist", "raw velocity"="Current/avg/speed", "distance units"=w195) -> ("correction factor"=w188:sgl, "strike velocity"=w189:sgl)  [unwired: 1 out]
            "DC_ factor" <- w188
            "Corrected Average" <- w189
            n110 = call "Velocity Correction.vi"("raw impact"="Current/impact/speed", "distance units"=w195, "raw redundant"="Current/redundant/speed", "raw residual"="Current/residual/speed", "screen set midpt to target"="Impac/Target Dist", "residual screen to target"="Residual/Target Dist", "correction coefficient"=w193) -> ("corrected impact"=w207:sgl, "corrected redundant"=w199:sgl, "corrected residual"=w205:sgl, "impact factor"=w202:sgl, "conversion factor"=→"conversion factor":sgl, "residual factor"=w201:sgl)  [unwired: 3 in]
            "Residual factor" <- w201
            "Impact factor" <- w202
            "Corrected Impact" <- w207
            "Corrected Residual" <- w205
            "Corrected Redundant" <- w199
            n111 = Not Equal?(x="Drag Corrected", y="old drag") -> (x != y?=w213:bool)
            n112 = Select(t=w199, s="Drag Corrected", f="Current/redundant/speed") -> (s? t:f=→"Redundant/speed":sgl)
            n113 = Select(t=w189, s="Drag Corrected", f="Current/avg/speed") -> (s? t:f=→"Avg/speed":sgl)
            n114 = Select(t=w207, s="Drag Corrected", f="Current/impact/speed") -> (s? t:f=→"Impact/speed":sgl)
            n115 = Select(t=w205, s="Drag Corrected", f="Current/residual/speed") -> (s? t:f=→"residual/speed":sgl)
            n116 = Not Equal?(x="Threat 2", y="old threat") -> (x != y?=w214:bool)
            n117 = Or(x=w214, y=w213) -> (x .or. y?=w212:bool)
            n118 = case shown="True" w212 {
              tunnel: "Threat 2" -> [_ w237]
              tunnel: w198 -> [w221 w236]
              tunnel: w201 -> [_ w235]
              tunnel: w202 -> [_ w234]
              tunnel: "Drag Corrected" -> [_ w233]
              tunnel: [w221 w232] -> w211
              tunnel: w188 -> [_ w222]
              frame False {
              }
              frame True {
                w223 = sgl 0.0  # sgl
                n119 = local write "old threat"(w237) -> ()
                n120 = property on="Threat 2" class="Ring (strict)"() -> ("Strings []"=w231:string[], "Value"=w230:u16)  [unwired: 2 in, 2 out]
                n121 = for {
                  tunnel: w236 -> [w244] mode=indexing
                  tunnel: w235 -> [w254]
                  tunnel: w234 -> [w249]
                  tunnel: w233 -> [w241]
                  tunnel: [w256] -> w232 mode=indexing
                  tunnel: w222 -> [w242]
                  n122 = Unbundle By Name(w244) -> ("Uncorrected Impact"=w248:sgl)
                  n123 = Unbundle By Name(w244) -> ("Uncorrected Residual"=w253:sgl)
                  n124 = Unbundle By Name(w244) -> ("UncorrectedRed_PB"=w251:sgl)
                  n125 = Unbundle By Name(w244) -> ("UncorrectedAvgVel_PB"=w243:sgl)
                  n126 = Multiply(x=w242, y=w243) -> (x*y=w239:sgl)
                  n127 = Multiply(x=w249, y=w251) -> (x*y=w250:sgl)
                  n128 = Multiply(x=w249, y=w248) -> (x*y=w246:sgl)
                  n129 = Multiply(x=w254, y=w253) -> (x*y=w245:sgl)
                  n130 = Select(t=w239, s=w241, f=w243) -> (s? t:f=w240:sgl)
                  n131 = Select(t=w250, s=w241, f=w251) -> (s? t:f=w252:sgl)
                  n132 = Select(t=w245, s=w241, f=w253) -> (s? t:f=w255:sgl)
                  n133 = Select(t=w246, s=w241, f=w248) -> (s? t:f=w247:sgl)
                  n134 = Subtract(x=w240, y=w239) -> (x-y=w238:sgl)
                  n135 = Bundle By Name(cluster=w244, "velLoss_PB"=w238, "strikeVel_PB"=w239, "avgVel_PB"=w240, "CorrectedRed_PB"=w250, "Redundant_Velocity"=w252, "Corrected Impact"=w246, "IMPACT VELOCITY"=w247, "Corrected residual"=w245, "RESIDUAL  VELOCITY"=w255) -> (w256:T4)
                }
                n136 = To Long Integer(number=w230) -> (32bit integer=w225:i32)
                n137 = Index Array(array=w231, index=w225) -> (element=w229:string)
                n138 = Scan From String(format string="%f " ("Format String"), input string=w229, default 1=w223) -> (output 1=w224:sgl)  [unwired: 2 in, 3 out]
                n139 = local write "old drag"(w233) -> ()
                n140 = Multiply(x=sgl 0.06479891, y=w224) -> (x*y=w226:sgl)
                n141 = local write "Projectile Mass"(w226) -> ()
              }
            }
            "SHOT STATUS" <- "Current/sthotstatus"
          }
          frame #3 {
            n142 = flat-sequence {
              tunnel: w261 -> [w265]
              tunnel: [w265] -> w260
              tunnel: w259 -> [w262]
              tunnel: [w262] -> w258
              tunnel: w260 -> [w274]
              tunnel: w258 -> [w272]
              tunnel: [w272] -> w257
              tunnel: w257 -> [w313]
              frame #0 {
                n143 = Array Size(array=w265) -> (size(s)=w271:i32)
                n144 = Array Size(array=w262) -> (size(s)=w267:i32)
                n145 = Equal To 0?(x=w271) -> (x = 0?=w263:bool)
                n146 = Equal To 0?(x=w267) -> (x = 0?=w264:bool)
                n147 = Or(x=w263, y=w264) -> (x .or. y?=w270:bool)
                n148 = Select(t=u8 2, s=w270, f=u8 0) -> (s? t:f=w266:u8)
                n149 = property on="String" class="Str"("Visible"=w264) -> ()  [unwired: 2 in, 2 out]
                n150 = property on="Save" class="Bool"("Disabled"=w266) -> ()  [unwired: 2 in, 2 out]
              }
              frame #1 {
                n151 = Array Size(array=w274) -> (size(s)=w273:i32)
                n152 = case shown="1, Default" w273 {
                  tunnel: w274 -> [_ w276]
                  frame 0 {
                  }
                  frame 1, Default {
                    w292 = sgl[] [] ("Partial")
                    # "This section calculates the V50"
                    n153 = for {
                      shift-right: [w302] -> w278
                      shift-left: w292 -> [w303]
                      shift-right: [w300] -> w277
                      shift-left: w292 -> [w301]
                      tunnel: w276 -> [w298] mode=indexing
                      tunnel: [w297] -> w275 mode=indexing
                      # "Here, DuPont uses:\n\nIMPACT VELOCITY"
                      n154 = Unbundle By Name(w298) -> ("avgVel_PB"=w297:sgl, "SHOT STATUS"=w299:u16)
                      n155 = case shown="0, Default" w299 {
                        tunnel: w297 -> [w304 w308]
                        tunnel: [w307 w309] -> w302
                        tunnel: w303 -> [w306 w309]
                        tunnel: w301 -> [w305 w311]
                        tunnel: [w305 w310] -> w300
                        frame 0, Default {
                          n156 = Build Array (concatenate)(w306, w304) -> (w307:sgl[])
                        }
                        frame 1 {
                          n157 = Build Array (concatenate)(w311, w308) -> (w310:sgl[])
                        }
                      }
                    }
                    n158 = Sort 1D Array(array=w278) -> (sorted array=w296:sgl[])
                    n159 = Sort 1D Array(array=w277) -> (sorted array=w283:sgl[])
                    "Complete" <- w283
                    n160 = Array Max & Min(array=w275) -> (max value=w287:sgl, min value=w286:sgl)  [unwired: 2 out]
                    n161 = Reverse 1D Array(array=w296) -> (reversed array=w281:sgl[])
                    "Partial" <- w281
                    n162 = Array Size(array=w283) -> (size(s)=→"number of completes":i32)
                    n163 = Array Max & Min(array=w283) -> (min value=w289:sgl)  [unwired: 3 out]
                    n164 = Array Size(array=w281) -> (size(s)=→"number of partials":i32)
                    n165 = Subtract(x=w287, y=w286) -> (x-y=w285:sgl)
                    n166 = Array Max & Min(array=w281) -> (max value=w291:sgl)  [unwired: 3 out]
                    n167 = To Long Integer(number=w289) -> (32bit integer=→"lowComplete":i32)
                    n168 = call "Compute V50.vi"("Maximum Deviation"="MaxDeviation", "Partial"=w281, "Complete"=w283) -> ("zmr"=→"Z.M.R.":sgl, "Points"=→"Pairs":i16, "V50"=→"computed_V50":sgl)
                    n169 = To Long Integer(number=w285) -> (32bit integer=→"rangeOfResults":i32)
                    n170 = To Long Integer(number=w291) -> (32bit integer=→"highPartial":i32)
                  }
                }
              }
              frame #2 {
                n171 = for {
                  tunnel: w313 -> [w322] mode=indexing
                  shift-right: [w319] -> w312
                  shift-left: u16 0 -> [w320]
                  n172 = Unbundle By Name(w322) -> ("Number of Plies"=w321:i32)
                  n173 = Greater Than 0?(x=w321) -> (x > 0?=w318:bool)
                  n174 = Select(t=u16 1 ("y"), s=w318, f=u16 0) -> (s? t:f=w315:u16)
                  n175 = Add(x=w320, y=w315) -> (x+y=w319:u16)
                }
                "plytypes" <- w312
              }
            }
          }
          frame #4 {
            # "This section plots  Impact velocity vs. loadingdata"
            n176 = Not(x="velocity-loading") -> (.not. x?=w329:bool)
            n177 = case shown="False" w329 {
              tunnel: "Powder" -> [w358 _]
              tunnel: "Earliest Date" -> [w360 _]
              tunnel: "Threat" -> [w359 _]
              tunnel: "latest Date" -> [w355 _]
              tunnel: w323 -> [w341 _]
              frame False {
                w337 = FALSE ("Visible")
                w338 = TRUE ("Visible")
                w361 = "" ("replace string (\"\")")
                n178 = invoke on="v50 data 2" class="Tbl" method="Reinit To Default"() -> (error out=w334:errorcluster)  [unwired: 3 in, 2 out]
                n179 = call "Trim String.vi"("inStr"=w358) -> ("outStr"=w356:string)
                n180 = call "Trim String.vi"("inStr"=w359) -> ("outStr"=w357:string)
                n181 = invoke on="Velocity versus Loading" class="XYGraph (strict)" method="Reinit To Default"(error in=w334) -> (error out=w333:errorcluster)  [unwired: 2 in, 2 out]
                n182 = property on="Data retrieval" class="Str"(error in=w333, "Visible"=w338, "Blinking"=w338) -> (error out=w335:errorcluster)  [unwired: 1 in, 1 out]
                n183 = Format Into String(format string="  select top %d experiment.threat,  shots.loading, shots.impact,  experiment.powder, shots.date from shots, experiment where shots.expt = experiment.expt and shots.loading > .02 and shots.date between  #%s# and #%s# and shots.impact between 5000 and 10 and experiment.powder like '%%%s%%' and experiment.threat like '%%%s%%' and experiment.threat<>'' order by experiment.threat, shots.loading,shots.impact" ("Format String"), error in=w335, "maxRecs", w360, w355, w356, w357) -> (resulting string=w365:string, error out=w331:errorcluster)  [unwired: 1 in]
                n184 = Search and Replace String(input string=w365, search string=" and experiment.powder like '%%'", replace string=w361, error in=w331) -> (result string=w363:string, error out=w332:errorcluster)  [unwired: 4 in, 2 out]
                n185 = Search and Replace String(input string=w363, search string="and experiment.threat like '%%'", replace string=w361, error in=w332) -> (result string=w342:string, error out=w330:errorcluster)  [unwired: 4 in, 2 out]
                n186 = call-poly <vilib>:"DB Tools Open Connection.vi"("error in (no error)"=w330, "connection information"=w341) -> ("error out"=w347:errorcluster, "connection reference"=w349:T9)  [unwired: 6 in]
                n187 = call-poly <vilib>:"DB Tools Execute Query.vi"("error in (no error)"=w347, "SQL query"=w342, "connection reference"=w349) -> ("error out"=w346:errorcluster, "recordset reference"=w350:T10)  [unwired: 5 in]
                n188 = call <vilib>:"DB Tools Fetch Table Data.vi"("error in (no error)"=w346, "recordset reference"=w350) -> ("error out"=w345:errorcluster, "recordset data"=w343:string[][], "recordset reference out"=w351:T10)  [unwired: 3 in]
                "v50 data 2" <- w343
                n189 = Array Size(array=w343) -> (size(s)=w353:i32[])
                n190 = Fract/Exp String To Number(string=w343) -> (number=w369:dbl[][])  [unwired: 3 in, 1 out]
                n191 = call-poly <vilib>:"DB Tools Free Object.vi"("error in (no error)"=w345, "recordset reference"=w351) -> ("error out"=w344:errorcluster, "connection reference"=w348:T9)  [unwired: 8 in]
                n192 = Index Array(array=w353) -> (element=→"ActualNumRecs":i32)  [unwired: 1 in]
                n193 = call <vilib>:"DB Tools Close Connection.vi"("error in (no error)"=w344, "connection reference"=w348) -> ("error out"=w340:errorcluster)  [unwired: 5 in]
                n194 = Index Array(array=w369, index (col)=2 ("Disabled Index (col)")) -> (element=w368:dbl[])  [unwired: 1 in]
                n195 = Index Array(array=w369, index (col)=1 ("Disabled Index (col)")) -> (element=w367:dbl[])  [unwired: 1 in]
                n196 = call "Continue DB Error Dialog.vi"("error in (no error)"=w340) -> ("error out"=w336:errorcluster)  [unwired: 3 in, 2 out]
                n197 = Bundle(w367, w368) -> (→"Velocity versus Loading":cluster{dbl[], dbl[]})  [unwired: 1 in]
                n198 = property on="Data retrieval" class="Str"(error in=w336, "Visible"=w337, "Blinking"=w337) -> ()  [unwired: 1 in, 2 out]
              }
              frame True {
              }
            }
          }
          frame #5 {
            # "This section plots panel V50 data"
            n199 = case shown="True" "Panel Search" {
              tunnel: w373 -> [_ w384]
              frame False {
              }
              frame True {
                n200 = invoke on="v50 data" class="Tbl" method="Reinit To Default"() -> (error out=w421:errorcluster)  [unwired: 3 in, 2 out]
                n201 = property on="queryThreat" class="Ring (strict)"() -> ("Strings []"=w419:string[], "Value"=w420:u16)  [unwired: 2 in, 2 out]
                n202 = invoke on="Previous V50 Data" class="WFGraph (strict)" method="Reinit To Default"(error in=w421) -> (error out=w422:errorcluster)  [unwired: 2 in, 2 out]
                n203 = To Long Integer(number=w420) -> (32bit integer=w378:i32)
                n204 = Index Array(array=w419, index=w378) -> (element=w415:string)
                n205 = Format Into String(format string="SELECT  Experiment.Date, Shots.impact\nFROM Shots, Experiment where Shots.Expt = Experiment.expt\nand Experiment.Date Between #%s# And #%s# AND Experiment.threat Like '%%%s%%'\nORDER BY Experiment.Date" ("SQL statement"), error in=w422, "DATE 2", "DATE 3", w415) -> (resulting string=w385:string, error out=w377:errorcluster)  [unwired: 1 in]
                n206 = call-poly <vilib>:"DB Tools Open Connection.vi"("error in (no error)"=w377, "connection information"=w384) -> ("error out"=w390:errorcluster, "connection reference"=w392:T9)  [unwired: 6 in]
                n207 = call-poly <vilib>:"DB Tools Execute Query.vi"("error in (no error)"=w390, "SQL query"=w385, "connection reference"=w392) -> ("error out"=w389:errorcluster, "recordset reference"=w393:T10)  [unwired: 5 in]
                n208 = call <vilib>:"DB Tools Fetch Table Data.vi"("error in (no error)"=w389, "recordset reference"=w393) -> ("error out"=w388:errorcluster, "recordset data"=w383:string[][], "recordset reference out"=w394:T10)  [unwired: 3 in]
                n209 = call-poly <vilib>:"DB Tools Free Object.vi"("error in (no error)"=w388, "recordset reference"=w394) -> ("error out"=w387:errorcluster, "connection reference"=w391:T9)  [unwired: 8 in]
                n210 = Array Size(array=w383) -> (size(s)=w414:i32[])
                n211 = Index Array(array=w414, index=0 ("Index")) -> (element=w412:i32)
                n212 = call <vilib>:"DB Tools Close Connection.vi"("error in (no error)"=w387, "connection reference"=w391) -> ("error out"=w386:errorcluster)  [unwired: 5 in]
                n213 = Decrement(x=w412) -> (x-1=w411:i32)
                n214 = call "Continue DB Error Dialog.vi"("error in (no error)"=w386) -> ("error out"=w376:errorcluster)  [unwired: 3 in, 2 out]
                n215 = Index Array(array=w383, index (row)=w411, index (col)=1 ("Disabled Index (col)")) -> (element=w410:string)
                n216 = Fract/Exp String To Number(string=w410) -> (number=w409:dbl)  [unwired: 3 in, 1 out]
                "Latest Velocity" <- w409
                n217 = Not Equal?(x=w410, y="" ("Empty String Constant")) -> (x != y?=w423:bool)
                n218 = Fract/Exp String To Number(string=w383) -> (number=w433:dbl[][])  [unwired: 3 in, 1 out]
                n219 = Select(t=w383, s=w423, f=string[][] [["", "NONE"], ["", ""]]) -> (s? t:f=→"v50 data":string[][])
                n220 = Index Array(array=w433, index (col)=1 ("Disabled Index (col)")) -> (element=w379:dbl[])  [unwired: 1 in]
                n221 = call <vilib>:"Std Deviation and Variance.vi"("X"=w379, "Weighting (Sample)"=enum16{"Sample", "Population"}."Sample") -> ("mean"=w381:dbl, "standard deviation"=w380:dbl)  [unwired: 1 out]
                "Average Velocity" <- w381
                "St. Deviation" <- w380
                n222 = Array Size(array=w379) -> (size(s)=w402:i32)
                n223 = Subtract(x=w381, y=w409) -> (x-y=w408:dbl)
                n224 = Absolute Value(x=w408) -> (abs(x)=w407:dbl)
                n225 = Multiply(x=3.0, y=w380) -> (x*y=w403:dbl)
                n226 = Divide(x=w407, y=w380) -> (x/y=w396:dbl)
                n227 = Subtract(x=w381, y=w403) -> (x-y=w400:dbl)
                n228 = Add(x=w381, y=w403) -> (x+y=w401:dbl)
                n229 = Initialize Array(w381, w402) -> (w432:dbl[])
                n230 = Initialize Array(w400, w402) -> (w399:dbl[])
                n231 = Initialize Array(w401, w402) -> (w398:dbl[])
                n232 = Format Into String(format string="%3.1f" ("Format String"), error in=w376, w396) -> (resulting string=w397:string, error out=w375:errorcluster)  [unwired: 1 in]
                n233 = Greater?(x=3.0, y=w396) -> (0:→"In Control":bool)
                n234 = Build Array(w379, w432, w399, w398) -> (w429:dbl[][])
                n235 = property on="In Control" class="Bool (strict)"(error in=w375, "Boolean Text.Text"=w397) -> (error out=w374:errorcluster)  [unwired: 1 in, 1 out]
                n236 = Bundle(0.0, 1.0, w429) -> (→"Previous V50 Data":cluster{dbl, dbl, dbl[][]})  [unwired: 1 in]
                n237 = call <vilib>:"Simple Error Handler.vi"("error in (no error)"=w374) -> ()  [unwired: 4 in, 5 out]
              }
            }
          }
          frame #6 {
            n238 = local read "Pairs"() -> (w443:i16)
            n239 = Sort 1D Array(array=w446) -> (sorted array=w447:T4[])
            n240 = for {
              tunnel: w447 -> [w506] mode=indexing
              tunnel: w443 -> [w497]
              shift-right: [w496] -> _
              shift-left: i16 0 -> [w495]
              tunnel: [w489] -> w436 mode=indexing
              # "this section marks the lowest completes that are used in V50"
              n241 = Unbundle By Name(w506) -> ("SHOT STATUS"=w493:u16, "Projectile Mass"=w491:sgl, "avgVel_PB"=w490:sgl, "RESIDUAL  VELOCITY"=w492:sgl)
              n242 = local read "conversion factor"() -> (w499:sgl)
              n243 = case shown="1" w493 {
                tunnel: w497 -> [_ w513]
                tunnel: [FALSE w512] -> w494
                tunnel: [w508 w511] -> w496
                tunnel: w495 -> [w508 w509]
                frame 0, Default {
                }
                frame 1 {
                  n244 = Less?(x=w509, y=w513) -> (x < y?=w512:bool)
                  n245 = Add(x=w509, y=i16 1 ("t")) -> (x+y=w511:i16)
                }
              }
              n246 = Multiply(x=w499, y=w492) -> (x*y=w500:sgl)
              n247 = Multiply(x=w490, y=w499) -> (x*y=w501:sgl)
              n248 = Multiply(x=w501, y=w501) -> (x*y=w505:sgl)
              n249 = Multiply(x=w500, y=w500) -> (x*y=w504:sgl)
              n250 = Subtract(x=w505, y=w504) -> (x-y=w503:sgl)
              n251 = Compound Arithmetic op=MULTIPLY(w491, w503, sgl 0.0005 ("Input")) -> (w498:sgl)
              n252 = Bundle By Name(cluster=w506, "usedv50"=w494, "Energy Loss (J)"=w498) -> (w489:T4)
            }
            n253 = Reverse 1D Array(array=w436) -> (reversed array=w442:T4[])
            n254 = for {
              tunnel: w442 -> [w468] mode=indexing
              tunnel: w443 -> [w471]
              shift-right: [w469] -> _
              shift-left: i16 0 -> [w470]
              tunnel: [w466] -> w437 mode=indexing
              # "chooses highest partials used in v50"
              n255 = Unbundle By Name(w468) -> ("SHOT STATUS"=w472:u16, "usedv50"=w465:bool)
              n256 = case shown="0, Default" w472 {
                tunnel: w471 -> [w476 _]
                tunnel: [w475 w479] -> w467
                tunnel: w470 -> [w473 w478]
                tunnel: [w474 w478] -> w469
                tunnel: w465 -> [_ w479]
                frame 0, Default {
                  n257 = Less?(x=w473, y=w476) -> (x < y?=w475:bool)
                  n258 = Add(x=w473, y=i16 1) -> (x+y=w474:i16)
                }
                frame 1 {
                }
              }
              n259 = Bundle By Name(cluster=w468, "usedv50"=w467) -> (w466:T4)
            }
            n260 = Not Equal?(x=w437, y="Old_Shots") -> (x != y?=w448:bool)
            n261 = Or(x="Reject shot", y="Delete Button") -> (x .or. y?=w458:bool)
            n262 = Or(x="RESET", y="reread") -> (x .or. y?=w463:bool)
            n263 = case shown="True" "Next Shot" {
              tunnel: w437 -> [_ w480]
              frame False {
              }
              frame True {
                n264 = property on="SHOTS" class="Arr (strict)"() -> ("Index Values"=w482:u32[])  [unwired: 2 in, 2 out]
                n265 = Array Size(array=w480) -> (size(s)=w485:i32)
                n266 = local write "Next Shot"(FALSE ("Boolean")) -> ()
                n267 = To Unsigned Long Integer(number=w485) -> (unsigned 32bit integer=w481:u32)
                n268 = Index Array(array=w482) -> (element=w487:u32)  [unwired: 1 in]
                n269 = Increment(x=w487) -> (x+1=w486:u32)
                n270 = Quotient & Remainder(x=w486, y=w481) -> (x-y*floor(x/y)=w484:u32)  [unwired: 1 out]
                n271 = Replace Array Subset(array=w482, new element=w484) -> (w483:u32[])  [unwired: 1 in]
                n272 = property on="SHOTS" class="Arr (strict)"("Index Values"=w483) -> ()  [unwired: 2 in, 2 out]
              }
            }
            n273 = case shown="True" w448 {
              tunnel: w437 -> [_ w514]
              frame False {
              }
              frame True {
                n274 = call "Sort Shots.vi"("shot array"=w514) -> ("shotTable OUT"=w515:string[][])
                n275 = local write "SHOTS"(w514) -> ()
                n276 = local write "Old_Shots"(w514) -> ()
                n277 = local write "Table of Shots"(w515) -> ()
              }
            }
            n278 = Build Array("EXIT", w463, "Report", "Save", "switch", "Accept Data", "RANGE RESET", w458, "Contact Shot Report", "Report_PB") -> (w451:bool[])
            n279 = Search 1D Array(1D array=w451, element=TRUE) -> (index of element=w450:i32)  [unwired: 1 in]
            n280 = case shown="True" "Stop Program" {
              frame False {
              }
              frame True {
                n281 = Stop() -> ()  [unwired: 1 in]
              }
            }
          }
        }
      }
      frame 0 {
        w517 = -1 ("index of element")
        # "This section stops program"
        n282 = Two Button Dialog(message="All Unsaved data will be lost.   Do you want to quit the program? ") -> (T button?=w519:bool)  [unwired: 2 in]
        n283 = case shown="True" w519 {
          frame False {
          }
          frame True {
            n284 = Quit LabVIEW(quit? (T)=TRUE) -> ()
          }
        }
      }
      frame 1 {
        # "This section reads the ini file"
        # "This section resets the entire program"
        n285 = case shown="0, Default" w525 {
          tunnel: [w528 TRUE] -> w526
          frame 0, Default {
            n286 = local read "RESET"() -> (w527:bool)
            n287 = case shown="True" w527 {
              tunnel: [TRUE w530] -> w528
              frame False {
              }
              frame True {
                n288 = Two Button Dialog(message="Reset will remove all unsaved data.  Do you want to RESET? ") -> (T button?=w530:bool)  [unwired: 2 in]
              }
            }
          }
          frame 100 {
          }
        }
        n289 = case shown="True" w526 {
          tunnel: w524 -> [_ w538]
          tunnel: w523 -> [_ w537]
          tunnel: [-1 ("index of element") w536] -> w522
          frame False {
            n290 = local write "RESET"(FALSE ("RESET")) -> ()
          }
          frame True {
            n291 = flat-sequence {
              tunnel: [w582] -> w535
              tunnel: w538 -> [w549]
              tunnel: w537 -> [w581]
              tunnel: [w611] -> w536
              tunnel: w535 -> [w611]
              frame #0 {
                # "New for PBBA"
                n292 = control-ref of="Panel Backing"() -> (w557:refnum<vi>)
                n293 = control-ref of="Submitter"() -> (w558:refnum<vi>)
                n294 = control-ref of="Panel Dimensions"() -> (w559:refnum<vi>)
                n295 = control-ref of="Powder Type"() -> (w560:refnum<vi>)
                n296 = control-ref of="Panel Type"() -> (w561:refnum<vi>)
                n297 = control-ref of="Method"() -> (w562:refnum<vi>)
                n298 = control-ref of="Panel Stitch"() -> (w563:refnum<vi>)
                n299 = control-ref of="ballistician"() -> (w568:refnum<vi>)
                n300 = control-ref of="Panel Technician"() -> (w567:refnum<vi>)
                n301 = control-ref of="Manufacturer"() -> (w566:refnum<vi>)
                n302 = control-ref of="Test Conditions"() -> (w565:refnum<vi>)
                n303 = control-ref of="Type"() -> (w564:refnum<vi>)
                n304 = call "Get INI Section.vi"("Ring Refnum"=w557, "configuration file path"=w549) -> ("error OUT"=w547:errorcluster)  [unwired: 4 in, 1 out]
                n305 = call "Get INI Section.vi"("Ring Refnum"=w558, "configuration file path"=w549) -> ("error OUT"=w546:errorcluster)  [unwired: 4 in, 1 out]
                n306 = call "Get INI Section.vi"("Ring Refnum"=w559, "configuration file path"=w549) -> ("error OUT"=w545:errorcluster)  [unwired: 4 in, 1 out]
                n307 = call "Get INI Section.vi"("Ring Refnum"=w560, "configuration file path"=w549) -> ("error OUT"=w544:errorcluster)  [unwired: 4 in, 1 out]
                n308 = call "Get INI Section.vi"("Ring Refnum"=w561, "configuration file path"=w549) -> ("error OUT"=w543:errorcluster)  [unwired: 4 in, 1 out]
                n309 = call "Get INI Section.vi"("Ring Refnum"=w562, "configuration file path"=w549) -> ("error OUT"=w542:errorcluster)  [unwired: 4 in, 1 out]
                n310 = call "Get INI Section.vi"("Ring Refnum"=w563, "configuration file path"=w549) -> ("error OUT"=w541:errorcluster)  [unwired: 4 in, 1 out]
                n311 = call "Get INI Section.vi"("Ring Refnum"=w568, "configuration file path"=w549) -> ()  [unwired: 4 in, 2 out]
                n312 = call "Get INI Section.vi"("Ring Refnum"=w567, "configuration file path"=w549) -> ()  [unwired: 4 in, 2 out]
                n313 = call "Get INI Section.vi"("Ring Refnum"=w566, "configuration file path"=w549) -> ()  [unwired: 4 in, 2 out]
                n314 = call "Get INI Section.vi"("Ring Refnum"=w565, "configuration file path"=w549) -> ()  [unwired: 4 in, 2 out]
                n315 = call "Get INI Section.vi"("Ring Refnum"=w564, "configuration file path"=w549) -> ("Array"=w574:string[])  [unwired: 4 in, 1 out]
                n316 = call "Read Parameters.vi"("appended path"=w549) -> ("midpt_to_target_dist"=w577:sgl, "max dev"=w587:sgl, "residual separation"=→"Residual/Separation":sgl, "impact separation"=→"Impact/Separation":sgl, "barrel screen dist"=→"Barrel to Screen Distance":sgl, "impact target dist"=w586:sgl, "resid target dist"=w585:sgl)  [unwired: 3 in]
                n317 = call "Read INI Section 2.vi"("section"="Threat with Correction Factor", "configuration file path"=w549) -> ("Array"=w593:string[])  [unwired: 4 in, 1 out]
                n318 = local write "Residual/Target Dist"(w585) -> ()
                n319 = local write "MaxDeviation"(w587) -> ()
                n320 = local write "Impac/Target Dist"(w586) -> ()
                n321 = local write "mid_to_targ_dist"(w577) -> ()
                n322 = Build Array(w547, w546, w545, w544, w543, w542, w541) -> (w540:errorcluster[])
                n323 = Insert Into Array "Insert Into Array"(array=w574, index=0 ("Index"), new element="ANY STYLE" ("New Element/Subarray")) -> (w548:string[])
                n324 = call "Split Factor Array.vi"("Split character"=":", "STRING INPUT"=w593) -> ("FACTOR OUTPUT"=→"factor array":sgl[], "STRING OUTPUT"=w591:string[])
                n325 = Merge Errors(w540) -> (w539:errorcluster)
                n326 = property on="Threat 2" class="Ring (strict)"("Strings []"=w591) -> ()  [unwired: 2 in, 2 out]
                n327 = property on="Ply Description" class="Ring (strict)"("Strings []"=w548) -> ()  [unwired: 2 in, 2 out]
                n328 = call <vilib>:"Simple Error Handler.vi"("error in (no error)"=w539) -> ()  [unwired: 4 in, 5 out]
                n329 = control-ref of="Fabric.vendor"() -> (w555:refnum<vi>)
                n330 = control-ref of="Fabric.styleNum"() -> (w556:refnum<vi>)
                n331 = control-ref of="Fabric.fiber"() -> (w550:refnum<vi>)
                n332 = control-ref of="Fabric.denier"() -> (w554:refnum<vi>)
                n333 = control-ref of="Fabric.pickWeave"() -> (w553:refnum<vi>)
                n334 = control-ref of="Fabric.finish"() -> (w552:refnum<vi>)
                n335 = control-ref of="Fabric.stitch"() -> (w551:refnum<vi>)
                n336 = control-ref of="covering"() -> (w569:refnum<vi>)
                n337 = control-ref of="shooter"() -> (w570:refnum<vi>)
                n338 = control-ref of="recorder"() -> (w571:refnum<vi>)
                n339 = control-ref of="weapon"() -> (w572:refnum<vi>)
                n340 = control-ref of="projectile"() -> (w573:refnum<vi>)
                n341 = call "Get INI Section.vi"("Ring Refnum"=w569, "configuration file path"=w549) -> ()  [unwired: 4 in, 2 out]
                n342 = call "Get INI Section.vi"("Ring Refnum"=w570, "configuration file path"=w549) -> ()  [unwired: 4 in, 2 out]
                n343 = call "Get INI Section.vi"("Ring Refnum"=w571, "configuration file path"=w549) -> ()  [unwired: 4 in, 2 out]
                n344 = call "Get INI Section.vi"("Ring Refnum"=w572, "configuration file path"=w549) -> ()  [unwired: 4 in, 2 out]
                n345 = call "Get INI Section.vi"("Ring Refnum"=w573, "configuration file path"=w549) -> ()  [unwired: 4 in, 2 out]
                n346 = call "Get INI Section.vi"("Ring Refnum"=w555, "configuration file path"=w549) -> ()  [unwired: 4 in, 2 out]
                n347 = call "Get INI Section.vi"("Ring Refnum"=w556, "configuration file path"=w549) -> ()  [unwired: 4 in, 2 out]
                n348 = call "Get INI Section.vi"("Ring Refnum"=w550, "configuration file path"=w549) -> ()  [unwired: 4 in, 2 out]
                n349 = call "Get INI Section.vi"("Ring Refnum"=w554, "configuration file path"=w549) -> ()  [unwired: 4 in, 2 out]
                n350 = call "Get INI Section.vi"("Ring Refnum"=w553, "configuration file path"=w549) -> ()  [unwired: 4 in, 2 out]
                n351 = call "Get INI Section.vi"("Ring Refnum"=w552, "configuration file path"=w549) -> ()  [unwired: 4 in, 2 out]
                n352 = call "Get INI Section.vi"("Ring Refnum"=w551, "configuration file path"=w549) -> ()  [unwired: 4 in, 2 out]
                n353 = invoke on="Stop Program" class="Bool (strict)" method="Reinit To Default"() -> ()  [unwired: 3 in, 3 out]
                n354 = local read "RESET"() -> (w584:bool)
                n355 = case shown="True" w584 {
                  tunnel: [errorcluster {"status"=FALSE, "code"=0, "source"=""} ("error out") w604] -> w583
                  tunnel: [-1 ("index of element") w600] -> w582
                  tunnel: w581 -> [_ w599]
                  frame False {
                  }
                  frame True {
                    n356 = local read "Data Source"() -> (w601:u16)
                    n357 = local write "RESET"(FALSE) -> ()
                    n358 = call "Get Last Record (SubVI).vi"("connect Str"=w599) -> ("shot record"=→"Shot":i32, "experiment record"=→"Panel":i32, "error out"=w604:errorcluster)
                    n359 = case shown="2" w601 {
                      tunnel: [-1 ("index of element") -1 ("index of element") 6 ("index of element")] -> w600
                      frame 0, Default {
                      }
                      frame 1 {
                      }
                      frame 2 {
                        # "check for\nPCI 6602"
                      }
                    }
                    n360 = invoke on="Complete" class="Arr (strict)" method="Reinit To Default"() -> ()  [unwired: 3 in, 3 out]
                    n361 = invoke on="Partial" class="Arr (strict)" method="Reinit To Default"() -> ()  [unwired: 3 in, 3 out]
                    n362 = invoke on="residual/speed" class="DigNum (strict)" method="Reinit To Default"() -> ()  [unwired: 3 in, 3 out]
                    n363 = invoke on="Pairs" class="DigNum (strict)" method="Reinit To Default"() -> ()  [unwired: 3 in, 3 out]
                    n364 = invoke on="Z.M.R." class="DigNum (strict)" method="Reinit To Default"() -> ()  [unwired: 3 in, 3 out]
                    n365 = invoke on="Impact/speed" class="DigNum (strict)" method="Reinit To Default"() -> ()  [unwired: 3 in, 3 out]
                    n366 = invoke on="computed_V50" class="DigNum (strict)" method="Reinit To Default"() -> ()  [unwired: 3 in, 3 out]
                    n367 = invoke on="Drag Corrected" class="Bool (strict)" method="Reinit To Default"() -> ()  [unwired: 3 in, 3 out]
                    n368 = invoke on="old drag" class="Bool (strict)" method="Reinit To Default"() -> ()  [unwired: 3 in, 3 out]
                    n369 = invoke on="Shot Decription" class="Str" method="Reinit To Default"() -> ()  [unwired: 3 in, 3 out]
                    n370 = invoke on="Save" class="Bool" method="Reinit To Default"() -> ()  [unwired: 3 in, 3 out]
                    n371 = invoke on="Accept Data" class="Bool (strict)" method="Reinit To Default"() -> ()  [unwired: 3 in, 3 out]
                    n372 = invoke on="old threat" class="DigNum (strict)" method="Reinit To Default"() -> ()  [unwired: 3 in, 3 out]
                    n373 = invoke on="Old_Shots" class="Arr (strict)" method="Reinit To Default"() -> ()  [unwired: 3 in, 3 out]
                    n374 = invoke on="SHOTS" class="Arr (strict)" method="Reinit To Default"() -> (error out=w602:errorcluster)  [unwired: 3 in, 2 out]
                    n375 = invoke on="Table of Shots" class="Tbl (strict)" method="Reinit To Default"(error in=w602) -> ()  [unwired: 2 in, 3 out]
                  }
                }
                n376 = Path To String(path=w549) -> (string=w588:string)
                n377 = case shown="False" "message control" {
                  tunnel: w583 -> [_ _]
                  tunnel: w588 -> [w595 _]
                  frame False {
                    n378 = local write "message control"(TRUE) -> ()
                    n379 = call "Ballistics Message Center.vi"("INI File Name"=w595) -> ()
                  }
                  frame True {
                  }
                }
              }
              frame #1 {
                n380 = One Button Dialog(message="Ballistic Test Program is now ready for use") -> ()  [unwired: 1 in, 1 out]
              }
            }
          }
        }
      }
      frame 2 {
        w667 = TRUE  # append on new line? (F)
        w707 = TRUE  # append on new line? (F)
        w739 = FALSE  # show grid lines
        w751 = -1 ("index of element")
        # "This section prepares a DuPont V50 report"
        # "add graph to 3rd box"
        n381 = invoke on="Shot Graph" class="XYGraph (strict)" method="Reinit To Default"() -> (error out=w720:errorcluster)  [unwired: 3 in, 2 out]
        n382 = property on="Submitter" class="Ring (strict)"() -> ("Strings []"=w654:string[], "Value"=w653:u16)  [unwired: 2 in, 2 out]
        n383 = control-ref of="Complete"() -> (w628:refnum<vi>)
        n384 = control-ref of="Points"() -> (w717:refnum<vi>)
        n385 = control-ref of="Partial"() -> (w716:refnum<vi>)
        n386 = To Long Integer(number=w653) -> (32bit integer=w627:i32)
        n387 = control-ref of="Value"() -> (w718:refnum<vi>)
        n388 = call "Graph V50.vi"("valueRef"=w718, "completeRef"=w628, "pointsRef"=w717, "partialRef"=w716, "error IN"=w720) -> ("shotGraph"=→"Shot Graph":cluster{i32[], sgl[]}[])
        n389 = Index Array(array=w654, index=w627) -> (element=w650:string)
        n390 = local read "Panel"() -> (w649:i32)
        n391 = call <vilib>:"New Report.vi"("report type"=T8."HTML", "error in (no error)"=w720) -> ("report out"=w741:refnum<class "NI_report.lvclass">, "error out"=w740:errorcluster)  [unwired: 12 in]
        n392 = Format Into String(format string="Serial Number: %5d<newline>Submitter: %s" ("Format String"), w649, w650) -> (resulting string=w648:string)  [unwired: 2 in, 1 out]
        n393 = call-dynamic "Set Report Font.vi"("report in"=w741, "text options"=T7 {"Italic"=enum."Italic Unchanged", "Strike Through"=enum."Strike Through Unchanged", "Underline"=enum."Underline Unchanged", "Bold"=enum."Bold On"}, "font settings"=T6 {"Charset (-1)"=-1, "Weight (-1)"=-1, "Name"="Arial", "Size"="4 "}, "error in (no error)"=w740) -> ("report out"=w725:refnum<class "NI_report.lvclass">, "error out"=w726:errorcluster)  [unwired: 9 in, 1 out]
        n394 = call-dynamic "Set Report Header Text.vi"("report in"=w725, "left header text"=w648, "center header text"="Ballistic V50 Report", "error in (no error)"=w726, "HTML header size"=enum16{"H1", "H2", "H3", "H4", "H5", "H6", "H7"}."H2") -> ("report out"=w728:refnum<class "NI_report.lvclass">, "error out"=w729:errorcluster)  [unwired: 9 in]
        n395 = local read "Room Temperature"() -> (w635:i32)
        n396 = local read "Fabric Description"() -> (w679:string)
        n397 = local read "Projectile Mass"() -> (w633:sgl)
        n398 = local read "Impact factor"() -> (w676:sgl)
        n399 = property on="Manufacturer" class="Ring (strict)"() -> ("Strings []"=w686:string[], "Value"=w685:u16)  [unwired: 2 in, 2 out]
        n400 = property on="Panel Backing" class="Ring (strict)"() -> ("Strings []"=w684:string[], "Value"=w683:u16)  [unwired: 2 in, 2 out]
        n401 = property on="Powder Type" class="Ring (strict)"() -> ("Strings []"=w682:string[], "Value"=w681:u16)  [unwired: 2 in, 2 out]
        n402 = property on="Threat 2" class="Ring (strict)"() -> ("Strings []"=w678:string[], "Value"=w677:u16)  [unwired: 2 in, 2 out]
        n403 = call-dynamic "Set Report Font.vi"("report in"=w728, "text options"=T7 {"Italic"=enum."Italic Unchanged", "Strike Through"=enum."Strike Through Unchanged", "Underline"=enum."Underline Unchanged", "Bold"=enum."Bold Off"}, "font settings"=T6 {"Charset (-1)"=-1, "Weight (-1)"=-1, "Name"="Arial", "Size"="1"}, "error in (no error)"=w729) -> ("report out"=w704:refnum<class "NI_report.lvclass">, "error out"=w705:errorcluster)  [unwired: 9 in, 1 out]
        n404 = Select(t="Disclosure on Ballistic and Stab Test Data<newline>The attached ballistic test data was generated by DuPont and corresponds to DuPont's current knowledge on the performance of the subject test panels against certain ballistic threats.  This information is offered solely to provide possible suggestions for your own experimentation and validation.  It is not intended as a substitute for your own testing or any testing you may need to submit for a bid package, you should undertake your own testing whether you do so yourself with the supplier of the materials to be tested or with an independent, third party, certified testing facility and the supplier of the materials to be tested (i.e., the fabric weaver).  DuPont makes no warranties, and assumes no liabilities in connection with any use of the information supplied with this disclosure statement." ("text"), s="Add Disclaimer", f="" ("t")) -> (s? t:f=w663:string)
        n405 = To Long Integer(number=w685) -> (32bit integer=w615:i32)
        n406 = To Long Integer(number=w683) -> (32bit integer=w618:i32)
        n407 = To Long Integer(number=w681) -> (32bit integer=w617:i32)
        n408 = To Long Integer(number=w677) -> (32bit integer=w616:i32)
        n409 = Index Array(array=w686, index=w615) -> (element=w680:string)
        n410 = call-poly <vilib>:"Append Report Text.vi"("report in"=w704, "text"=w663, "error in (no error)"=w705) -> ("report out"=w703:refnum<class "NI_report.lvclass">, "error out"=w701:errorcluster)  [unwired: 9 in, 2 out]
        n411 = Index Array(array=w684, index=w618) -> (element=w632:string)
        n412 = Index Array(array=w682, index=w617) -> (element=w670:string)
        n413 = Index Array(array=w678, index=w616) -> (element=w638:string)
        n414 = property on="Test Conditions" class="Ring (strict)"() -> ("Strings []"=w675:string[], "Value"=w674:u16)  [unwired: 2 in, 2 out]
        n415 = property on="Panel Type" class="Ring (strict)"() -> ("Strings []"=w673:string[], "Value"=w672:u16)  [unwired: 2 in, 2 out]
        n416 = local read "Z.M.R."() -> (w661:sgl)
        n417 = call-dynamic "Set Report Font.vi"("report in"=w703, "text options"=T7 {"Italic"=enum."Italic Unchanged", "Strike Through"=enum."Strike Through Unchanged", "Underline"=enum."Underline Unchanged", "Bold"=enum."Bold Unchanged"}, "font settings"=T6 {"Charset (-1)"=-1, "Weight (-1)"=-1, "Name"="Arial", "Size"="3 "}, "error in (no error)"=w701) -> ("report out"=w702:refnum<class "NI_report.lvclass">, "error out"=w700:errorcluster)  [unwired: 9 in, 1 out]
        n418 = local read "Room Humidity"() -> (w637:i32)
        n419 = local read "Weight of Panel"() -> (w634:dbl)
        n420 = local read "Sample ID"() -> (w630:string)
        n421 = local read "Areal Density"() -> (w631:dbl)
        n422 = local read "Shot Angle"() -> (w669:u16)
        n423 = call-dynamic "New Report Line.vi"("report in"=w702, "error in (no error)"=w700) -> ("report out"=w742:refnum<class "NI_report.lvclass">, "error out"=w743:errorcluster)  [unwired: 12 in]
        n424 = To Long Integer(number=w674) -> (32bit integer=w614:i32)
        n425 = To Long Integer(number=w672) -> (32bit integer=w613:i32)
        n426 = Index Array(array=w675, index=w614) -> (element=w668:string)
        n427 = call-dynamic "New Report Line.vi"("report in"=w742, "error in (no error)"=w743) -> ("report out"=w709:refnum<class "NI_report.lvclass">, "error out"=w708:errorcluster)  [unwired: 12 in]
        n428 = Index Array(array=w673, index=w613) -> (element=w636:string)
        n429 = Format Into String(format string="<table border=\"0\" cellspacing=\"6\"><tr><td align=\"left\"><b>Fabric Parameters</b></td><td>&nbsp;</td><td>&nbsp;</td><td align=\"left\"><b>Test Parameters</b></td><td>&nbsp;</td></tr><tr><td align=\"right\">Sample ID: </td><td align=\"left\">%s</td><td>&nbsp;</td><td align=\"right\">Method: </td><td align=\"left\">V50</td></tr><tr><td align=\"right\">Areal Density: </td><td align=\"left\">%.3f</td><td>&nbsp;</td><td align=\"right\">Threat: </td><td align=\"left\">%s</td></tr><tr><td align=\"right\">Manufacturer: </td><td align=\"left\">%s</td><td>&nbsp;</td><td align=\"right\">Room Temperature: </td><td align=\"left\">%.0f</td></tr><tr><td align=\"right\">Group Data: </td><td align=\"left\">%s</td><td>&nbsp;</td><td align=\"right\">Correction Factor: </td><td align=\"left\">%0.4f</td></tr><tr><td align=\"right\">Projectile Weight: </td><td align=\"left\">%0.3f</td><td>&nbsp;</td><td align=\"right\">Panel Backing: </td><td align=\"left\">%s</td></tr><tr><td align=\"right\">Powder Type: </td><td align=\"left\">%s</td><td>&nbsp;</td><td align=\"right\">Shot Angle: </td><td align=\"left\">%.0f</td></tr><tr><td align=\"right\">Test Conditions: </td><td align=\"left\">%s</td><td>&nbsp;</td><td align=\"right\">Room Humidity: </td><td align=\"left\">%.0f</td></tr><tr><td align=\"right\">Panel Weight: </td><td align=\"left\">%.4f</td><td>&nbsp;</td><td>&nbsp;</td></tr><tr><td align=\"right\">Descripton: </td><td align=\"left\">%s</td><td>&nbsp;</td><td>&nbsp;</td></tr></table>", w630, w631, w638, w680, w635, w679, w676, w633, w632, w670, w669, w668, w637, w634, w636) -> (resulting string=w665:string)  [unwired: 2 in, 1 out]
        n430 = property on="ballistician" class="Ring (strict)"() -> ("Strings []"=w690:string[], "Value"=w689:u16)  [unwired: 2 in, 2 out]
        n431 = call-poly <vilib>:"Append Report Text.vi"("report in"=w709, "text"=w665, "append on new line? (F)"=w707, "error in (no error)"=w708) -> ("report out"=w642:refnum<class "NI_report.lvclass">, "error out"=w643:errorcluster)  [unwired: 8 in, 2 out]
        n432 = To Long Integer(number=w689) -> (32bit integer=w612:i32)
        n433 = call-dynamic "New Report Line.vi"("report in"=w642, "error in (no error)"=w643) -> ("report out"=w736:refnum<class "NI_report.lvclass">, "error out"=w737:errorcluster)  [unwired: 12 in]
        n434 = local read "computed_V50"() -> (w706:sgl)
        n435 = Get Date/Time String(date format (0)=enum16{"short", "long", "abbreviated"}."abbreviated") -> (date string=w697:string)  [unwired: 2 in, 1 out]
        n436 = Index Array(array=w690, index=w612) -> (element=w688:string)
        n437 = local read "Sample ID"() -> (w652:string)
        n438 = property on="Table of Shots" class="Tbl (strict)"() -> ("Column Header Strings[]"=w719:string[])  [unwired: 2 in, 2 out]
        n439 = Less Than 0?(x=w661) -> (x < 0?=w662:bool)
        n440 = call-dynamic "New Report Line.vi"("report in"=w736, "error in (no error)"=w737) -> ("report out"=w735:refnum<class "NI_report.lvclass">, "error out"=w734:errorcluster)  [unwired: 12 in]
        n441 = Concatenate Strings(w697, " © " ("right footer text"), "  DuPont ") -> (w713:string)
        n442 = local read "Pairs"() -> (w687:i16)
        n443 = Select(t="Low Complete-High Partial: ", s=w662, f="Zone of Mixed Results: ") -> (s? t:f=w657:string)
        n444 = Format Value(format string="Panel %s.html  " ("string (\"\")"), value (0)=w652) -> (output string=w712:string)  [unwired: 1 in]
        n445 = call-poly <vilib>:"Append Table to Report.vi"("report in"=w735, "column width (1)"=1.1, "column headers"=w719, "text data"="Table of Shots", "error in (no error)"=w734, "show grid lines"=w739) -> ("report out"=w691:refnum<class "NI_report.lvclass">, "error out"=w695:errorcluster)  [unwired: 6 in, 2 out]
        n446 = Build Path(base path="Report Path", name or relative path=w712) -> (appended path=w710:path)
        n447 = Concatenate Strings(" V50:  %10.1f<newline>Number of Pairs Used: %d<newline>  ", w657, "%.1f<newline><newline>Ballistician:%s<newline> ") -> (w655:string)
        n448 = Format Into String(format string=w655, w706, w687, w661, w688) -> (resulting string=w626:string)  [unwired: 2 in, 1 out]
        n449 = call-dynamic "Set Report Font.vi"("report in"=w691, "text options"=T7 {"Italic"=enum."Italic Unchanged", "Strike Through"=enum."Strike Through Unchanged", "Underline"=enum."Underline On", "Bold"=enum."Bold Off"}, "font settings"=T6 {"Charset (-1)"=-1, "Weight (-1)"=-1, "Name"="Arial", "Size"="3 "}, "error in (no error)"=w695) -> ("report out"=w692:refnum<class "NI_report.lvclass">, "error out"=w693:errorcluster)  [unwired: 9 in, 1 out]
        n450 = call-dynamic "New Report Line.vi"("report in"=w692, "error in (no error)"=w693) -> ("report out"=w733:refnum<class "NI_report.lvclass">, "error out"=w732:errorcluster)  [unwired: 12 in]
        n451 = control-ref of="Shot Graph"() -> (w666:refnum<vi>)
        n452 = call-poly <vilib>:"Append Report Text.vi"("report in"=w733, "text"=w626, "append on new line? (F)"=w667, "error in (no error)"=w732) -> ("report out"=w640:refnum<class "NI_report.lvclass">, "error out"=w639:errorcluster)  [unwired: 8 in, 2 out]
        n453 = call-dynamic "Append Control Image to Report.vi"("report in"=w640, "image file type (.jpg)"=enum16{".jpg", ".png"}.".jpg" ("image file type(.png)"), "ctrl reference"=w666, "description"="Graph of Test Results" ("control name"), "error in (no error)"=w639) -> ("report out"=w625:refnum<class "NI_report.lvclass">, "error out"=w624:errorcluster)  [unwired: 7 in, 2 out]
        n454 = call-dynamic "Set Report Footer Text.vi"("report in"=w625, "right footer text"=w713, "error in (no error)"=w624) -> ("report out"=w730:refnum<class "NI_report.lvclass">, "error out"=w731:errorcluster)  [unwired: 11 in]
        n455 = call-dynamic "Get Report Type.vi"("report in"=w730, "error in (no error)"=w731) -> ("report out"=w747:refnum<class "NI_report.lvclass">, "report type"=w746:T8, "error out"=w750:errorcluster)  [unwired: 11 in]
        n456 = case shown="\"Standard Report\", Default" w746 {
          tunnel: w747 -> [w756 w761 w763 w765]
          tunnel: [w755 w760 w763 w765] -> w748
          tunnel: [w754 w759 w762 w764] -> w749
          tunnel: w750 -> [w753 w758 w762 w764]
          tunnel: w710 -> [_ w757 _ _]
          frame "Standard Report", Default {
            n457 = call-dynamic "Print Report.vi"("report in"=w756, "error in (no error)"=w753) -> ("report out"=w755:refnum<class "NI_report.lvclass">, "error out"=w754:errorcluster)  [unwired: 12 in]
          }
          frame "HTML" {
            n458 = call-dynamic "Save Report to File.vi"("report in"=w761, "report file path"=w757, "error in (no error)"=w758) -> ("report out"=w760:refnum<class "NI_report.lvclass">, "error out"=w759:errorcluster)  [unwired: 11 in]
          }
          frame "Word" {
          }
          frame "Excel" {
          }
        }
        n459 = call-dynamic "Dispose Report.vi"("report in"=w748, "error in (no error)"=w749) -> ("error out"=w644:errorcluster)  [unwired: 13 in]
        n460 = call <vilib>:"Simple Error Handler.vi"("error in (no error)"=w644) -> ("error out"=w645:errorcluster)  [unwired: 4 in, 4 out]
        n461 = case shown="No Error" w645 {
          frame No Error {
            n462 = One Button Dialog(message="A V50 Report is ready.") -> ()  [unwired: 1 in, 1 out]
          }
          frame Error {
          }
        }
      }
      frame 3 {
        # "This section saves the shots to the data base"
        n463 = stacked-sequence {
          seq-local: [w776 _ _] -> [_ w940 _]
          seq-local: [w775 _ _] -> [_ w934 _]
          seq-local: [_ w920 _] -> [_ _ w952]
          seq-local: [_ w922 _] -> [_ _ w951]
          seq-local: [_ w918 _] -> [_ _ w944]
          seq-local: [w787 _ _] -> [_ w917 _]
          seq-local: [w786 _ _] -> [_ w916 _]
          tunnel: w772 -> [_ _ w953]
          tunnel: [_ _ w946] -> w767
          tunnel: [_ _ w949] -> w771
          tunnel: w770 -> [w785 _ _]
          tunnel: w768 -> [w777 _ _]
          frame #0 {
            n464 = local read "fab1_totalWt"() -> (w784:sgl)
            n465 = local read "fab2_totalWt"() -> (w783:sgl)
            n466 = local read "fab3_totalWt"() -> (w782:sgl)
            n467 = local read "fab4_totalWt"() -> (w781:sgl)
            n468 = local read "fab5_totalWt"() -> (w780:sgl)
            n469 = local read "fab6_totalWt"() -> (w779:sgl)
            n470 = Array Size(array=w777) -> (size(s)=w791:i32)
            n471 = Format Into String(format string=" VALUES (%d ", w791) -> (resulting string=w790:string)  [unwired: 2 in, 1 out]
            n472 = Build Array(w784, w783, w782, w781, w780, w779) -> (w778:sgl[])
            n473 = for {
              tunnel: w777 -> [w842] mode=indexing
              shift-right: [w835] -> w775
              shift-left: w790 -> [w837]
              shift-right: [w831] -> w776
              shift-left: "insert into experiment (plytypes " ("SQL statement") -> [w832]
              tunnel: w778 -> [w793] mode=indexing
              i -> [w834]
              n474 = Unbundle By Name(w842) -> ("Number of Plies"=w795:i32, "Layer Comments"=w838:string, "Ply Description"=w840:u16, "Fabric.vendor"=w827:u16, "Fabric.styleNum"=w817:u16, "Fabric.fiber"=w816:u16, "Fabric.denier"=w815:u16, "Fabric.pickWeave"=w814:u16, "Fabric.finish"=w811:u16, "LotNum"=w809:string, "RollNum"=w810:string, "ozPerYd2"=w794:sgl, "Fabric.stitch"=w798:u16)
              n475 = Increment(x=w834) -> (x+1=w792:i32)
              n476 = Format Into String(format string=", ply%1dnumber, ply%1dtext, fab%1d_vendor_PB, fab%1d_styleNum_PB, fab%1d_fiberType_PB, fab%1d_denier_PB, fab%1d_pickWeave_PB, fab%1d_finishType_PB, fab%1d_lotNum_PB, fab%1d_rollNum_PB, fab%1d_ozPerYd2_PB,fab%1d_stitch_PB, fab%1d_totalWeight_PB", initial string=w832, w792, w792, w792, w792, w792, w792, w792, w792, w792, w792, w792, w792, w792) -> (resulting string=w831:string)  [unwired: 1 in, 1 out]
              n477 = To Long Integer(number=w840) -> (32bit integer=w830:i32)
              n478 = To Long Integer(number=w827) -> (32bit integer=w829:i32)
              n479 = To Long Integer(number=w817) -> (32bit integer=w822:i32)
              n480 = To Long Integer(number=w816) -> (32bit integer=w823:i32)
              n481 = To Long Integer(number=w815) -> (32bit integer=w821:i32)
              n482 = To Long Integer(number=w814) -> (32bit integer=w820:i32)
              n483 = To Long Integer(number=w811) -> (32bit integer=w812:i32)
              n484 = To Long Integer(number=w798) -> (32bit integer=w799:i32)
              n485 = property on="Fabric.stitch" class="Ring (strict)"() -> ("Strings []"=w796:string[])  [unwired: 2 in, 2 out]
              n486 = property on="Ply Description" class="Ring (strict)"() -> ("Strings []"=w828:string[])  [unwired: 2 in, 2 out]
              n487 = property on="Fabric.styleNum" class="Ring (strict)"() -> ("Strings []"=w824:string[])  [unwired: 2 in, 2 out]
              n488 = property on="Fabric.denier" class="Ring (strict)"() -> ("Strings []"=w819:string[])  [unwired: 2 in, 2 out]
              n489 = property on="Fabric.vendor" class="Ring (strict)"() -> ("Strings []"=w826:string[])  [unwired: 2 in, 2 out]
              n490 = property on="Fabric.fiber" class="Ring (strict)"() -> ("Strings []"=w825:string[])  [unwired: 2 in, 2 out]
              n491 = property on="Fabric.pickWeave" class="Ring (strict)"() -> ("Strings []"=w818:string[])  [unwired: 2 in, 2 out]
              n492 = property on="Fabric.finish" class="Ring (strict)"() -> ("Strings []"=w813:string[])  [unwired: 2 in, 2 out]
              n493 = Index Array(array=w828, index=w830) -> (element=w839:string)
              n494 = Index Array(array=w826, index=w829) -> (element=w803:string)
              n495 = Index Array(array=w824, index=w822) -> (element=w804:string)
              n496 = Index Array(array=w825, index=w823) -> (element=w805:string)
              n497 = Index Array(array=w819, index=w821) -> (element=w806:string)
              n498 = Index Array(array=w818, index=w820) -> (element=w807:string)
              n499 = Index Array(array=w813, index=w812) -> (element=w808:string)
              n500 = Index Array(array=w796, index=w799) -> (element=w797:string)
              n501 = call <vilib>:"Space Constant.vi"() -> ("String"=w800:string)
              n502 = Concatenate Strings(w838, "   " ("Substring"), w839) -> (w836:string)
              n503 = Concatenate Strings(w809, w800) -> (w802:string)
              n504 = Concatenate Strings(w810, w800) -> (w801:string)
              n505 = Format Into String(format string=", %d,  '%s',  '%s',  '%s',  '%s',  '%s',  '%s',  '%s',  '%s',  '%s', %.1f,  '%s', %.2f ", initial string=w837, w795, w836, w803, w804, w805, w806, w807, w808, w802, w801, w794, w797, w793) -> (resulting string=w835:string)  [unwired: 1 in, 1 out]
            }
            n506 = call-poly <vilib>:"DB Tools Open Connection.vi"("connection information"=w785) -> ("error out"=w786:errorcluster, "connection reference"=w787:T9)  [unwired: 7 in]
          }
          frame #1 {
            w932 = " " ("Substring")
            # "DP/PB shared requirements:"
            # "Added PBBA requirements:"
            n507 = local read "Panel"() -> (w919:i32)
            n508 = local read "currentDateTime"() -> (w941:string)
            n509 = local read "computed_V50"() -> (w930:sgl)
            n510 = local read "Drag Corrected"() -> (w925:bool)
            n511 = local read "Impact factor"() -> (w927:sgl)
            n512 = local read "Shot Angle"() -> (w943:u16)
            n513 = Increment(x=w919) -> (x+1=w918:i32)
            n514 = control-ref of="ballistician"() -> (w856:refnum<vi>)
            n515 = control-ref of="Submitter"() -> (w855:refnum<vi>)
            n516 = control-ref of="Test Conditions"() -> (w854:refnum<vi>)
            n517 = control-ref of="Type"() -> (w861:refnum<vi>)
            n518 = control-ref of="Panel Stitch"() -> (w862:refnum<vi>)
            n519 = control-ref of="Panel Type"() -> (w863:refnum<vi>)
            n520 = control-ref of="Threat 2"() -> (w865:refnum<vi>)
            n521 = control-ref of="weight(gr)"() -> (w845:refnum<vi>)
            n522 = local read "Total Number of Layers"() -> (w913:i32)
            n523 = local read "SHOTS"() -> (w942:T4[])
            n524 = call "Dropdown Selection (SubVI).vi"("reference"=w856) -> ("element"=w853:string)
            n525 = call "Dropdown Selection (SubVI).vi"("reference"=w855) -> ("element"=w852:string)
            n526 = call "Dropdown Selection (SubVI).vi"("reference"=w854) -> ("element"=w851:string)
            n527 = call "Dropdown Selection (SubVI).vi"("reference"=w861) -> ("element"=w860:string)
            n528 = call "Dropdown Selection (SubVI).vi"("reference"=w862) -> ("element"=w859:string)
            n529 = call "Dropdown Selection (SubVI).vi"("reference"=w863) -> ("element"=w858:string)
            n530 = call "Dropdown Selection (SubVI).vi"("reference"=w865) -> ("element"=w864:string)
            n531 = call "Dropdown Selection (SubVI).vi"("reference"=w845) -> ("element"=w844:string)
            n532 = Select(t=w927, s=w925, f=sgl 1.0) -> (s? t:f=w926:sgl)
            n533 = Concatenate Strings(w860, w932, w859, w932, w858, w932, "Fabric Description") -> (w905:string)
            n534 = local read "zmr 2"() -> (w907:sgl)
            n535 = control-ref of="Manufacturer"() -> (w879:refnum<vi>)
            n536 = control-ref of="Powder Type"() -> (w877:refnum<vi>)
            n537 = control-ref of="Panel Backing"() -> (w875:refnum<vi>)
            n538 = control-ref of="N.I.J"() -> (w873:refnum<vi>)
            n539 = control-ref of="Method"() -> (w871:refnum<vi>)
            n540 = control-ref of="Panel Dimensions"() -> (w869:refnum<vi>)
            n541 = control-ref of="Panel Technician"() -> (w867:refnum<vi>)
            n542 = Array Size(array=w942) -> (size(s)=w914:i32)
            n543 = Divide(x=w930, y=w926) -> (x/y=w929:sgl)
            n544 = call "Dropdown Selection (SubVI).vi"("reference"=w879) -> ("element"=w878:string)
            n545 = call "Dropdown Selection (SubVI).vi"("reference"=w877) -> ("element"=w876:string)
            n546 = call "Dropdown Selection (SubVI).vi"("reference"=w875) -> ("element"=w874:string)
            n547 = call "Dropdown Selection (SubVI).vi"("reference"=w873) -> ("element"=w872:string)
            n548 = call "Dropdown Selection (SubVI).vi"("reference"=w871) -> ("element"=w870:string)
            n549 = call "Dropdown Selection (SubVI).vi"("reference"=w869) -> ("element"=w868:string)
            n550 = call "Dropdown Selection (SubVI).vi"("reference"=w867) -> ("element"=w866:string)
            n551 = local read "highPartial"() -> (w850:i32)
            n552 = local read "totalBAW"() -> (w857:sgl)
            n553 = local read "rangeOfResults"() -> (w848:i32)
            n554 = control-ref of="standard"() -> (w904:refnum<vi>)
            n555 = control-ref of="workType"() -> (w900:refnum<vi>)
            n556 = control-ref of="covering"() -> (w895:refnum<vi>)
            n557 = control-ref of="shooter"() -> (w892:refnum<vi>)
            n558 = control-ref of="recorder"() -> (w890:refnum<vi>)
            n559 = control-ref of="rangeNum"() -> (w847:refnum<vi>)
            n560 = control-ref of="weapon"() -> (w885:refnum<vi>)
            n561 = control-ref of="projectile"() -> (w881:refnum<vi>)
            n562 = control-ref of="barrelLen"() -> (w880:refnum<vi>)
            n563 = call "Dropdown Selection (SubVI).vi"("reference"=w904) -> ("element"=w903:string)
            n564 = call "Dropdown Selection (SubVI).vi"("reference"=w900) -> ("element"=w899:string)
            n565 = call "Dropdown Selection (SubVI).vi"("reference"=w895) -> ("element"=w894:string)
            n566 = call "Dropdown Selection (SubVI).vi"("reference"=w892) -> ("element"=w891:string)
            n567 = call "Dropdown Selection (SubVI).vi"("reference"=w890) -> ("element"=w889:string)
            n568 = call "Dropdown Selection (SubVI).vi"("reference"=w847) -> ("element"=w846:string)
            n569 = call "Dropdown Selection (SubVI).vi"("reference"=w885) -> ("element"=w884:string)
            n570 = call "Dropdown Selection (SubVI).vi"("reference"=w881) -> ("element"=w883:string)
            n571 = call "Dropdown Selection (SubVI).vi"("reference"=w880) -> ("element"=w882:string)
            n572 = local read "lowComplete"() -> (w849:i32)
            n573 = Format Into String(format string=", %d, #%s#, '%s', '%s', %d, '%s', '%s', %.4f, '%s', '%s', '%s', %.4f, %.1f, %.6f, '%s', %.4f, '%s', %d, '%s', %d, '%s', '%s', %d, '%s', %d, %d, %.2f, '%s', %.1f, '%s', '%s', '%s', '%s', '%s', '%s', '%s', '%s', %.1f, %.1f, '%s', %d, '%s', '%s', '%s', '%s', '%s', '%s', %.1f, '%s', %.1f, %d, %d, %d)" ("Format String"), initial string=w934, w918, w941, w853, w852, w943, w851, w905, "Areal Density", "Areal density text", w864, w844, "Weight of Panel", w930, w929, w878, "Thickness", w876, w914, w874, w913, "Test Comments", w872, "B.F.S (mm)", w870, "Room Temperature", "Room Humidity", "Version", w868, w907, "Sample ID", w866, w903, "projName", "projNum", w899, "serialNum", "modelNum", "totalSampleWt", w857, w894, "minV50", w891, w889, w846, w884, w883, w882, "clayTemp", "clayCalib", "clayAverage", w850, w849, w848) -> (resulting string=w933:string)  [unwired: 1 in, 1 out]
            n574 = Concatenate Strings(w940, ", expt, [date], operator, submitter, angle, conditions, fabric, density, densitytext, threat,weight, panelweight, v50dc, v50 , maker, thickness, powder, numshots, backing, totalnumberplys, testcomments, nij, bfs, method, temperature, humidity, version, dimensions, zmr, sampleid, panelmaker,\nstandard_PB, projName_PB, projNum_PB, workType_PB, serialNum_PB, model_PB, totalSampleWt_PB,totalBAW_PB,covering_PB, minV50_PB,  shooter_PB, recorder_PB, rangeNum_PB, weapon_PB, projectile_PB, barrelLen_PB, clayTemp_PB, clayCal_PB, clayAvg_PB, highPartial_PB, lowComplete_PB, rangeOfResults_PB)" ("Substring"), w933) -> (w924:string)
            n575 = call-poly <vilib>:"DB Tools Execute Query.vi"("error in (no error)"=w916, "SQL query"=w924, "connection reference"=w917) -> ("error out"=w923:errorcluster, "recordset reference"=w921:T10)  [unwired: 5 in]
            n576 = call-poly <vilib>:"DB Tools Free Object.vi"("error in (no error)"=w923, "recordset reference"=w921) -> ("error out"=w922:errorcluster, "connection reference"=w920:T9)  [unwired: 8 in]
          }
          frame #2 {
            # "Experiment.expt"
            n577 = local read "Shot"() -> (w950:i32)
            n578 = Increment(x=w950) -> (x+1=w948:i32)
            n579 = for {
              tunnel: w953 -> [w997] mode=indexing
              tunnel: w952 -> [w969]
              tunnel: w951 -> [w971]
              tunnel: [w967] -> w945
              tunnel: [w968] -> w947
              tunnel: w948 -> [w975]
              tunnel: [w966] -> w949
              tunnel: w944 -> [w962]
              i -> [w966]
              # "Shot.id"
              n580 = Add(x=w975, y=w966) -> (x+y=w974:i32)
              n581 = Unbundle By Name(w997) -> ("IMPACT VELOCITY"=w983:sgl, "Redundant_Velocity"=w958:sgl, "RESIDUAL  VELOCITY"=w957:sgl, "Shot Description"=w959:string, "Powder Loading"=w987:sgl, "Barrel Temperature"=w988:sgl, "TIME / DATE"=w989:string, "shot order"=w990:i32, "Shot Angle"=w991:u16, "BackFace\nDepth"=w992:sgl, "BackFace\nDiameter"=w993:sgl, "SHOT STATUS"=w995:u16, "Projectile Mass"=w986:sgl, "usedv50"=w985:bool, "Energy Loss (J)"=w984:sgl, "avgVel_PB"=w965:sgl, "velLoss_PB"=w964:sgl, "strikeVel_PB"=w963:sgl)
              n582 = local read "Drag Corrected"() -> (w955:bool)
              n583 = local read "Residual factor"() -> (w980:sgl)
              n584 = local read "Impact factor"() -> (w954:sgl)
              n585 = Select(t=w954, s=w955, f=sgl 1.0) -> (s? t:f=w978:sgl)
              n586 = Select(t=w954, s=w955, f=sgl 1.0) -> (s? t:f=w960:sgl)
              n587 = Select(t=w980, s=w955, f=sgl 1.0) -> (s? t:f=w979:sgl)
              n588 = Greater Than 0?(x=w995) -> (x > 0?=w994:bool)
              n589 = Divide(x=w983, y=w978) -> (x/y=w976:sgl)
              n590 = Divide(x=w958, y=w960) -> (x/y=w956:sgl)
              n591 = Divide(x=w957, y=w979) -> (x/y=w982:sgl)
              n592 = Format Into String(format string="INSERT INTO shots (impactdc, redundantdc, residualdc,  comment, loading, barreltemp, [date], [order], shotangle, bfdepth, bfdiameter, [complete], expt, id, weight,usedv50, loss, residual, impact, redundant, avgVel_PB, velLoss_PB, strikeVel_PB)  VALUES (%.1f, %.1f, %.1f, '%s', %.4f, %.1f, #%s#, %d, %d, %.3f, %.3f, %d, %d, %d, %.4f, %d, %.4f, %.1f, %.1f, %.1f, %.1f, %.1f, %.1f)" ("Substring"), w983, w958, w957, w959, w987, w988, w989, w990, w991, w992, w993, w994, w962, w974, w986, w985, w984, w982, w976, w956, w965, w964, w963) -> (resulting string=w970:string)  [unwired: 2 in, 1 out]
              n593 = call-poly <vilib>:"DB Tools Execute Query.vi"("error in (no error)"=w971, "SQL query"=w970, "connection reference"=w969) -> ("error out"=w973:errorcluster, "recordset reference"=w972:T10)  [unwired: 5 in]
              n594 = call-poly <vilib>:"DB Tools Free Object.vi"("error in (no error)"=w973, "recordset reference"=w972) -> ("error out"=w967:errorcluster, "connection reference"=w968:T9)  [unwired: 8 in]
            }
            n595 = call <vilib>:"DB Tools Close Connection.vi"("error in (no error)"=w945, "connection reference"=w947) -> ("error out"=w946:errorcluster)  [unwired: 5 in]
          }
        }
        n596 = case shown="No Error" w767 {
          selector: w767 -> [w999 w1017]
          tunnel: [100 w1019] -> w773
          tunnel: [1 w1019] -> w774
          tunnel: w771 -> [w1012 _]
          tunnel: w766 -> [w1000 _]
          frame No Error {
            w1001 = "Data Base Parameters" ("section")
            n597 = local read "Shot"() -> (w1013:i32)
            n598 = call <vilib>:"Open Config Data (compatibility).vi"("error in (no error)"=w999, "configuration file path"=w1000) -> ("error out"=w1005:errorcluster, "refnum"=w1004:T11)  [unwired: 7 in, 1 out]
            n599 = Increment(x=w1013) -> (x+1=w1007:i32)
            n600 = Add(x=w1007, y=w1012) -> (x+y=w1008:i32)
            n601 = local write "Shot"(w1008) -> ()
            n602 = local read "Panel"() -> (w1009:i32)
            n603 = call-poly <vilib>:"Write Key.vi"("section"=w1001, "error in (no error)"=w1005, "value"=w1008, "key"="Last Shot Saved ", "refnum"=w1004) -> ("error out"=w1003:errorcluster, "refnum out"=w1002:T11)  [unwired: 4 in, 1 out]
            n604 = Increment(x=w1009) -> (x+1=w1006:i32)
            n605 = flat-sequence {
              tunnel: w998 -> [_]
              frame #0 {
                n606 = One Button Dialog(message="Data Saved") -> ()  [unwired: 1 in, 1 out]
              }
            }
            n607 = local write "Panel"(w1006) -> ()
            n608 = call-poly <vilib>:"Write Key.vi"("section"=w1001, "error in (no error)"=w1003, "value"=w1006, "key"="Last Panel Saved ", "refnum"=w1002) -> ()  [unwired: 4 in, 3 out]
            n609 = call <vilib>:"Close Config Data.vi"("error in (no error)"=w1003, "refnum"=w1002) -> ("error out"=w998:errorcluster)  [unwired: 8 in, 1 out]
          }
          frame Error {
            w1019 = -1
            n610 = call <vilib>:"Simple Error Handler.vi"("error in (no error)"=w1017) -> ()  [unwired: 4 in, 5 out]
            n611 = One Button Dialog(message="Error saving Data. ") -> ()  [unwired: 1 in, 1 out]
          }
        }
      }
      frame 4 {
        w1032 = -1 ("index of element")
        # "This section is supposed to switch the setting from partial to complete"
        n612 = Array Size(array=w1022) -> (size(s)=w1031:i32)
        n613 = Decrement(x=w1031) -> (x-1=w1023:i32)
        n614 = Index Array(array=w1022, index=w1023) -> (element=w1026:T4)
        n615 = Unbundle By Name(w1026) -> ("SHOT STATUS"=w1030:u16)
        n616 = Equal To 0?(x=w1030) -> (x = 0?=w1029:bool)
        n617 = Select(t=u16 1, s=w1029, f=u16 0) -> (s? t:f=w1025:u16)
        n618 = local write "Current/sthotstatus"(w1025) -> ()
        n619 = Bundle By Name(cluster=w1026, "SHOT STATUS"=w1025) -> (w1024:T4)
        n620 = Replace Array Subset(array=w1022, new element=w1024, index=w1023) -> (w1021:T4[])
        n621 = stacked-sequence {
          tunnel: w1025 -> [_]
          tunnel: w1021 -> [w1033]
          frame #0 {
            n622 = call "Sort Shots.vi"("shot array"=w1033) -> ("shotTable OUT"=w1034:string[][])
            n623 = local write "Table of Shots"(w1034) -> ()
            n624 = local write "SHOTS"(w1033) -> ()
          }
        }
      }
      frame 5 {
        w1074 = -1 ("index of element")
        # "Shot Order"
        # "This section accepts new data"
        n625 = local read "residual/speed"() -> (w1047:sgl)
        n626 = local read "Impact/speed"() -> (w1042:sgl)
        n627 = property on="Reject shot" class="Bool"("Disabled"=u8 0) -> ()  [unwired: 2 in, 2 out]
        n628 = local read "Current/redundant/speed"() -> (w1040:sgl)
        n629 = local read "Current/residual/speed"() -> (w1064:sgl)
        n630 = local read "Current/impact/speed"() -> (w1039:sgl)
        n631 = local write "Accept Data"(FALSE) -> ()
        n632 = local read "BACKFACE DIAMETER"() -> (w1069:sgl)
        n633 = local read "Corrected Redundant"() -> (w1037:sgl)
        n634 = local read "Current/avg/speed"() -> (w1035:sgl)
        n635 = local read "Corrected Residual"() -> (w1065:sgl)
        n636 = Array Size(array=w1061) -> (size(s)=w1067:i32)
        n637 = local read "BACKFACE DEPTH"() -> (w1060:sgl)
        n638 = local read "Redundant/speed"() -> (w1038:sgl)
        n639 = local read "Corrected Impact"() -> (w1063:sgl)
        n640 = local read "conversion factor"() -> (w1052:sgl)
        n641 = local read "SHOT STATUS"() -> (w1068:u16)
        n642 = local read "Avg/speed"() -> (w1036:sgl)
        n643 = Increment(x=w1067) -> (x+1=w1041:i32)
        n644 = Multiply(x=w1042, y=w1052) -> (x*y=w1054:sgl)
        n645 = Multiply(x=w1052, y=w1047) -> (x*y=w1053:sgl)
        n646 = Multiply(x=w1054, y=w1054) -> (x*y=w1059:sgl)
        n647 = Multiply(x=w1053, y=w1053) -> (x*y=w1058:sgl)
        n648 = Subtract(x=w1059, y=w1058) -> (x-y=w1056:sgl)
        n649 = Format Date/Time String(time format string (%c)="%x   %H:%M:%S") -> (date/time string=w1046:string)  [unwired: 2 in]
        "SUBMIT DATE/TIME" <- w1046
        n650 = Compound Arithmetic op=MULTIPLY("Projectile Mass", w1056, sgl 0.0005 ("Input")) -> (w1051:sgl)
        n651 = Index Array(array=w1061) -> (element=w1070:T4)  [unwired: 1 in]
        n652 = Bundle By Name(cluster=w1070, "TIME / DATE"=w1046, "shot order"=w1041, "IMPACT VELOCITY"=w1042, "RESIDUAL  VELOCITY"=w1047, "Shot Description"="Shot Decription", "Powder Loading"="Powder Loading", "Barrel Temperature"="Barrel Temp", "SHOT STATUS"=w1068, "BackFace\nDepth"=w1060, "BackFace\nDiameter"=w1069, "Shot Angle"="Shot Angle", "Uncorrected Impact"=w1039, "Corrected Impact"=w1063, "Uncorrected Residual"=w1064, "Corrected residual"=w1065, "Projectile Mass"="Projectile Mass", "Energy Loss (J)"=w1051, "UncorrectedRed_PB"=w1040, "Redundant_Velocity"=w1038, "CorrectedRed_PB"=w1037, "UncorrectedAvgVel_PB"=w1035, "avgVel_PB"=w1036) -> (w1066:T4)
        n653 = Build Array (concatenate)(w1061, w1066) -> (w1049:T4[])
        n654 = call "Sort Shots.vi"("shot array"=w1049) -> ("shotTable OUT"=w1050:string[][])
        n655 = local write "Table of Shots"(w1050) -> ()
        n656 = local write "SHOTS"(w1049) -> ()
      }
      frame 6 {
        w1082 = -1
        # "This section will reset range"
        n657 = Concatenate Strings(w1078, "6|") -> (w1075:string)
        n658 = case shown="2" "Data Source" {
          tunnel: [w1083 w1084 w1087] -> w1077
          tunnel: w1076 -> [w1083 w1084 w1086]
          tunnel: w1075 -> [_ _ w1085]
          frame 0, Default {
          }
          frame 1 {
          }
          frame 2 {
            w1095 = u32 22 items=["NI-DAQ version", "device name", "base address", "data transfer mode for analog input", "data transfer mode for analog output group 1", "data transfer mode for analog output group 2", "data transfer mode for GPCTR 0", "data transfer mode for GPCTR 1", "data transfer mode for digital I/O group 1", "data transfer mode for digital I/O group 2", "device type code", "DMA A level", "DMA B level", "DMA C level", "interrupt A level", "interrupt B level", "reserved", "lpt device mode", "DAQCard-700 counter 1 source", "interrupt generation mode", "device state during suspend mode", "computer name", "serial number", "counter type", "Scarab A Memory Size", "Scarab B Memory Size"] ("information type")
            w1094 = u32 1  # device
            # "Screens"
            n659 = Concatenate Strings(w1085, "2|") -> (w1090:string)
            n660 = call "Get DAQ Device Information.vi"("information type"=w1095, "task ID or device"=w1094) -> ("error out"=w1089:errorcluster, "information string"=w1093:string)  [unwired: 7 in, 1 out]
            n661 = disable-structure "Diagram Disable Structure" shown="Disabled" {
              disable-tunnel: w1090 -> [w1101 _]
              disable-tunnel: w1089 -> [w1098 w1103]
              disable-tunnel: [w1097 w1103] -> w1088
              frame Disabled {
                n662 = Current VI's Path() -> (path=w1102:path)
                n663 = call "Where Am I (SubVI).vi"("TL Calling Location"=w1101, "Call VI path"=w1102) -> ("I'm here"=w1100:string)
                n664 = call "Error Check (SubVI).vi"("calling VI"=w1100, "tag #"=0, "error IN"=w1098) -> ("error OUT"=w1097:errorcluster)  [unwired: 2 in]
              }
              frame Enabled {
                # "Debug code is disabled"
              }
            }
            n665 = Unbundle By Name(w1089) -> ("status"=w1096:bool)
            n666 = case shown="False" w1096 {
              tunnel: w1093 -> [w1112 _]
              tunnel: [w1112 "DEVICE NOT READY!" ("information string")] -> w1092
              tunnel: w1088 -> [w1111 _]
              tunnel: [w1104 w1117] -> w1087
              tunnel: w1086 -> [_ w1117]
              frame False {
                # "assign task IDs to counters"
                n667 = call "Config Counter to Measure Two Edge Separation.vi"("error IN"=w1111, "Counter"="Impact Timer", "device"="DAQ Card") -> ("error out"=w1114:errorcluster, "task ID out"=w1107:u32)  [unwired: 1 in]
                "impact/ID" <- w1107
                n668 = call "Config Counter to Measure Two Edge Separation.vi"("error IN"=w1114, "Counter"="Residual  Timer", "device"="DAQ Card") -> ("error out"=w1116:errorcluster, "task ID out"=w1105:u32)  [unwired: 1 in]
                "residual/ID" <- w1105
                n669 = call "Config Counter to Measure Two Edge Separation.vi"("error IN"=w1116, "Counter"="Redundant Timer", "device"="DAQ Card") -> ("error out"=w1115:errorcluster, "task ID out"=w1106:u32)  [unwired: 1 in]
                "Red/ID" <- w1106
                n670 = Bundle("task ID out"=w1107, "task ID out"=w1106, "task ID out"=w1105) -> (w1104:T12)  [unwired: 1 in]
                n671 = call <vilib>:"Simple Error Handler.vi"("error in (no error)"=w1115) -> ()  [unwired: 4 in, 5 out]
              }
              frame True {
                w1120 = u16 0 items=["Simulated", "Radar", "Screens"] ("Data Source")
                n672 = local write "Data Source"(w1120) -> ()
                n673 = One Button Dialog(message="Error initializing Timer board.  Switching to simulation") -> ()  [unwired: 1 in, 1 out]
              }
            }
            "Device S/N" <- w1092
          }
        }
        n674 = local write "SUBMIT DATE/TIME"("" ("Empty String Constant")) -> ()
      }
      frame 7 {
        w1126 = -1
        # "This section unaccepts new data  OR deletes the currently accessed previous shot"
        n675 = local read "Delete Button"() -> (w1125:bool)
        n676 = case shown="True" w1125 {
          tunnel: w1124 -> [w1129 w1141]
          tunnel: [w1130 w1142] -> w1122
          frame False {
            n677 = Array Size(array=w1129) -> (size(s)=w1127:i32)
            n678 = local write "SUBMIT DATE/TIME"("" ("Empty String Constant")) -> ()
            n679 = while {
              tunnel: [w1133] -> w1128
              tunnel: w1127 -> [w1135]
              tunnel: w1129 -> [w1137] mode=indexing
              i -> [w1133]
              stop <- w1136 stop-if-true
              n680 = Unbundle By Name(w1137) -> ("shot order"=w1134:i32)
              n681 = Equal?(x=w1134, y=w1135) -> (x = y?=w1136:bool)
            }
            n682 = Delete From Array "Delete From Array"(array=w1129, index=w1128) -> (array with subset deleted=w1130:T4[])  [unwired: 1 in, 1 out]
            n683 = property on="Reject shot" class="Bool"("Disabled"=u8 2) -> ()  [unwired: 2 in, 2 out]
          }
          frame True {
            n684 = property on="SHOTS" class="Arr (strict)"() -> ("Index Values"=w1150:u32[])  [unwired: 2 in, 2 out]
            n685 = Index Array(array=w1150, index=0 ("Index")) -> (element=w1140:u32)
            n686 = local write "Delete Button"(FALSE) -> ()
            n687 = Index Array(array=w1141, index=w1140) -> (element=w1139:T4)
            n688 = Unbundle By Name(w1139) -> ("shot order"=w1138:i32)
            n689 = Format Into String(format string="The currently displayed Shot, #%d", w1138) -> (resulting string=w1147:string)  [unwired: 2 in, 1 out]
            n690 = Concatenate Strings(w1147, ", will be deleted.  IT CANNOT RECOVERED!  Do you want to DELETE the shot?" ("message")) -> (w1146:string)
            n691 = Two Button Dialog(message=w1146, 1:"NO I do NOT want to delete.  Cancel Request" ("F button name (\"Cancel\")"), 2:"YES I want to delete the shot" ("T button name (\"OK\")")) -> (T button?=w1153:bool)
            n692 = case shown="True" w1153 {
              tunnel: w1141 -> [w1166 w1169]
              tunnel: [w1166 w1171] -> w1144
              tunnel: w1140 -> [_ w1168]
              tunnel: [10000 ("shot order") w1170] -> w1143
              frame False {
              }
              frame True {
                n693 = Index Array(array=w1169, index=w1168) -> (element=w1167:T4)
                n694 = Unbundle By Name(w1167) -> ("shot order"=w1170:i32)
                n695 = Delete From Array(array=w1169, index=w1168) -> (array with subset deleted=w1171:T4[])  [unwired: 1 in, 1 out]
              }
            }
            n696 = for {
              tunnel: [w1160] -> w1142 mode=indexing
              tunnel: w1144 -> [w1155] mode=indexing
              tunnel: w1143 -> [w1159]
              n697 = Unbundle By Name(w1155) -> ("shot order"=w1157:i32)
              n698 = Decrement(x=w1157) -> (x-1=w1156:i32)
              n699 = Greater?(x=w1157, y=w1159) -> (0:w1158:bool)
              n700 = case shown="True" w1158 {
                tunnel: w1156 -> [_ w1163]
                tunnel: w1155 -> [w1161 w1164]
                tunnel: [w1161 w1162] -> w1160
                frame False {
                }
                frame True {
                  n701 = Bundle By Name(cluster=w1164, "shot order"=w1163) -> (w1162:T4)
                }
              }
            }
          }
        }
        n702 = call "Sort Shots.vi"("shot array"=w1122) -> ("shotTable OUT"=w1123:string[][])
        n703 = local write "Table of Shots"(w1123) -> ()
        n704 = local write "SHOTS"(w1122) -> ()
      }
      frame 8 {
        w1177 = 0.0 ("Input 1")
        w1187 = "TBD" ("Input 2")
        w1197 = TRUE  # append on new line? (F)
        w1210 = TRUE  # append on new line? (F)
        w1234 = FALSE  # show grid lines
        w1244 = -1 ("index of element")
        # "This section prepares a Contact Shot report"
        # "add graph to 3rd box"
        n705 = call <vilib>:"New Report.vi"("report type"=T8."HTML") -> ("report out"=w1236:refnum<class "NI_report.lvclass">, "error out"=w1235:errorcluster)  [unwired: 13 in]
        n706 = call-dynamic "Set Report Font.vi"("report in"=w1236, "text options"=T7 {"Italic"=enum."Italic Unchanged", "Strike Through"=enum."Strike Through Unchanged", "Underline"=enum."Underline Unchanged", "Bold"=enum."Bold On"}, "font settings"=T6 {"Charset (-1)"=-1, "Weight (-1)"=-1, "Name"="Arial", "Size"="4 "}, "error in (no error)"=w1235) -> ("report out"=w1220:refnum<class "NI_report.lvclass">, "error out"=w1221:errorcluster)  [unwired: 9 in, 1 out]
        n707 = call-dynamic "Set Report Header Text.vi"("report in"=w1220, "center header text"="PBBA Ballistic CONTACT SHOT Report ", "error in (no error)"=w1221, "HTML header size"=enum16{"H1", "H2", "H3", "H4", "H5", "H6", "H7"}."H1") -> ("report out"=w1223:refnum<class "NI_report.lvclass">, "error out"=w1224:errorcluster)  [unwired: 10 in]
        n708 = call-dynamic "Set Report Font.vi"("report in"=w1223, "text options"=T7 {"Italic"=enum."Italic Unchanged", "Strike Through"=enum."Strike Through Unchanged", "Underline"=enum."Underline Unchanged", "Bold"=enum."Bold Off"}, "font settings"=T6 {"Charset (-1)"=-1, "Weight (-1)"=-1, "Name"="Arial", "Size"="1"}, "error in (no error)"=w1224) -> ("report out"=w1208:refnum<class "NI_report.lvclass">, "error out"=w1209:errorcluster)  [unwired: 9 in, 1 out]
        n709 = call-poly <vilib>:"Append Report Text.vi"("report in"=w1208, "text"="Disclosure on Ballistic and Stab Test Data<newline>The attached ballistic test data was generated by PBBA and corresponds to PBBA's current knowledge on the performance of the subject test panels against certain ballistic threats.  This information is offered solely to provide possible suggestions for your own experimentation and validation.  It is not intended as a substitute for your own testing or any testing you may need to submit for a bid package, you should undertake your own testing whether you do so yourself with the supplier of the materials to be tested or with an independent, third party, certified testing facility and the supplier of the materials to be tested (i.e., the fabric weaver).  PBBA makes no warranties, and assumes no liabilities in connection with any use of the information supplied with this disclosure statement.", "error in (no error)"=w1209) -> ("report out"=w1207:refnum<class "NI_report.lvclass">, "error out"=w1205:errorcluster)  [unwired: 9 in, 2 out]
        n710 = call-dynamic "Set Report Font.vi"("report in"=w1207, "text options"=T7 {"Italic"=enum."Italic Unchanged", "Strike Through"=enum."Strike Through Unchanged", "Underline"=enum."Underline Unchanged", "Bold"=enum."Bold Unchanged"}, "font settings"=T6 {"Charset (-1)"=-1, "Weight (-1)"=-1, "Name"="Arial", "Size"="3 "}, "error in (no error)"=w1205) -> ("report out"=w1206:refnum<class "NI_report.lvclass">, "error out"=w1204:errorcluster)  [unwired: 9 in, 1 out]
        n711 = call-dynamic "New Report Line.vi"("report in"=w1206, "error in (no error)"=w1204) -> ("report out"=w1237:refnum<class "NI_report.lvclass">, "error out"=w1238:errorcluster)  [unwired: 12 in]
        n712 = local read "Sample ID"() -> (w1176:string)
        n713 = call-dynamic "New Report Line.vi"("report in"=w1237, "error in (no error)"=w1238) -> ("report out"=w1212:refnum<class "NI_report.lvclass">, "error out"=w1211:errorcluster)  [unwired: 12 in]
        n714 = Format Into String(format string="<table border=\"0\" cellspacing=\"6\"><tr><td align=\"left\"><b>Fabric Parameters</b></td><td>&nbsp;</td><td>&nbsp;</td><td align=\"left\"><b>Test Parameters</b></td><td>&nbsp;</td></tr><tr><td align=\"right\">Sample ID: </td><td align=\"left\">%s</td><td>&nbsp;</td><td align=\"right\">Method: </td><td align=\"left\">V50</td></tr><tr><td align=\"right\">Areal Density: </td><td align=\"left\">%.3f</td><td>&nbsp;</td><td align=\"right\">Threat: </td><td align=\"left\">%s</td></tr><tr><td align=\"right\">Manufacturer: </td><td align=\"left\">%s</td><td>&nbsp;</td><td align=\"right\">Room Temperature: </td><td align=\"left\">%.0f</td></tr><tr><td align=\"right\">Group Data: </td><td align=\"left\">%s</td><td>&nbsp;</td><td align=\"right\">Correction Factor: </td><td align=\"left\">%0.4f</td></tr><tr><td align=\"right\">Projectile Weight: </td><td align=\"left\">%0.3f</td><td>&nbsp;</td><td align=\"right\">Panel Backing: </td><td align=\"left\">%s</td></tr><tr><td align=\"right\">Powder Type: </td><td align=\"left\">%s</td><td>&nbsp;</td><td align=\"right\">Shot Angle: </td><td align=\"left\">%.0f</td></tr><tr><td align=\"right\">Test Conditions: </td><td align=\"left\">%s</td><td>&nbsp;</td><td align=\"right\">Room Humidity: </td><td align=\"left\">%.0f</td></tr><tr><td align=\"right\">Panel Weight: </td><td align=\"left\">%.4f</td><td>&nbsp;</td><td>&nbsp;</td></tr><tr><td align=\"right\">Descripton: </td><td align=\"left\">%s</td><td>&nbsp;</td><td>&nbsp;</td></tr></table>", w1176, w1177, w1187, w1187, w1177, w1187, w1177, w1177, w1187, w1187, w1177, w1187, w1177, w1177, w1187) -> (resulting string=w1196:string)  [unwired: 2 in, 1 out]
        n715 = call-poly <vilib>:"Append Report Text.vi"("report in"=w1212, "text"=w1196, "append on new line? (F)"=w1210, "error in (no error)"=w1211) -> ("report out"=w1191:refnum<class "NI_report.lvclass">, "error out"=w1192:errorcluster)  [unwired: 8 in, 2 out]
        n716 = call-dynamic "New Report Line.vi"("report in"=w1191, "error in (no error)"=w1192) -> ("report out"=w1231:refnum<class "NI_report.lvclass">, "error out"=w1232:errorcluster)  [unwired: 12 in]
        n717 = local read "Sample ID"() -> (w1178:string)
        n718 = call-dynamic "New Report Line.vi"("report in"=w1231, "error in (no error)"=w1232) -> ("report out"=w1230:refnum<class "NI_report.lvclass">, "error out"=w1229:errorcluster)  [unwired: 12 in]
        n719 = local read "Report Path"() -> (w1179:path)
        n720 = call-poly <vilib>:"Append Table to Report.vi"("report in"=w1230, "column width (1)"=1.1, "text data"=string[][] [["TBD"]], "error in (no error)"=w1229, "show grid lines"=w1234) -> ("report out"=w1198:refnum<class "NI_report.lvclass">, "error out"=w1202:errorcluster)  [unwired: 7 in, 2 out]
        n721 = Format Value(format string="SHOT %s.html  " ("string (\"\")"), value (0)=w1178) -> (output string=w1215:string)  [unwired: 1 in]
        n722 = Build Path(base path=w1179, name or relative path=w1215) -> (appended path=w1213:path)
        n723 = call-dynamic "Set Report Font.vi"("report in"=w1198, "text options"=T7 {"Italic"=enum."Italic Unchanged", "Strike Through"=enum."Strike Through Unchanged", "Underline"=enum."Underline On", "Bold"=enum."Bold Off"}, "font settings"=T6 {"Charset (-1)"=-1, "Weight (-1)"=-1, "Name"="Arial", "Size"="3 "}, "error in (no error)"=w1202) -> ("report out"=w1199:refnum<class "NI_report.lvclass">, "error out"=w1200:errorcluster)  [unwired: 9 in, 1 out]
        n724 = control-ref of="Shot Graph"() -> (w1183:refnum<vi>)
        n725 = call-dynamic "New Report Line.vi"("report in"=w1199, "error in (no error)"=w1200) -> ("report out"=w1228:refnum<class "NI_report.lvclass">, "error out"=w1227:errorcluster)  [unwired: 12 in]
        n726 = call-poly <vilib>:"Append Report Text.vi"("report in"=w1228, "append on new line? (F)"=w1197, "error in (no error)"=w1227) -> ("report out"=w1189:refnum<class "NI_report.lvclass">, "error out"=w1188:errorcluster)  [unwired: 9 in, 2 out]
        n727 = call-dynamic "Append Control Image to Report.vi"("report in"=w1189, "image file type (.jpg)"=enum16{".jpg", ".png"}.".jpg" ("image file type(.png)"), "ctrl reference"=w1183, "description"="Graph of Test Results" ("control name"), "error in (no error)"=w1188) -> ("report out"=w1173:refnum<class "NI_report.lvclass">, "error out"=w1174:errorcluster)  [unwired: 7 in, 2 out]
        n728 = call-dynamic "Set Report Footer Text.vi"("report in"=w1173, "error in (no error)"=w1174) -> ("report out"=w1225:refnum<class "NI_report.lvclass">, "error out"=w1226:errorcluster)  [unwired: 12 in]
        n729 = call-dynamic "Get Report Type.vi"("report in"=w1225, "error in (no error)"=w1226) -> ("report out"=w1240:refnum<class "NI_report.lvclass">, "report type"=w1239:T8, "error out"=w1243:errorcluster)  [unwired: 11 in]
        n730 = case shown="\"HTML\"" w1239 {
          tunnel: w1240 -> [w1249 w1254 w1255 w1258]
          tunnel: [w1248 w1253 w1255 w1258] -> w1241
          tunnel: [w1247 w1252 w1256 w1257] -> w1242
          tunnel: w1243 -> [w1246 w1251 w1256 w1257]
          tunnel: w1213 -> [_ w1250 _ _]
          frame "Standard Report", Default {
            n731 = call-dynamic "Print Report.vi"("report in"=w1249, "error in (no error)"=w1246) -> ("report out"=w1248:refnum<class "NI_report.lvclass">, "error out"=w1247:errorcluster)  [unwired: 12 in]
          }
          frame "HTML" {
            n732 = call-dynamic "Save Report to File.vi"("report in"=w1254, "report file path"=w1250, "error in (no error)"=w1251) -> ("report out"=w1253:refnum<class "NI_report.lvclass">, "error out"=w1252:errorcluster)  [unwired: 11 in]
          }
          frame "Word" {
          }
          frame "Excel" {
          }
        }
        n733 = call-dynamic "Dispose Report.vi"("report in"=w1241, "error in (no error)"=w1242) -> ("error out"=w1193:errorcluster)  [unwired: 13 in]
        n734 = call <vilib>:"Simple Error Handler.vi"("error in (no error)"=w1193) -> ("error out"=w1194:errorcluster)  [unwired: 4 in, 4 out]
        n735 = case shown="No Error" w1194 {
          frame No Error {
            n736 = One Button Dialog(message="A CONTACT SHOT Report is ready.") -> ()  [unwired: 1 in, 1 out]
          }
          frame Error {
          }
        }
      }
      frame 9 {
        w1284 = TRUE  # Enable
        w1289 = -1 ("index of element")
        # "Create DHB Ballistic Test Report"
        n737 = stacked-sequence {
          tunnel: [_ w1346 _] -> w1275
          tunnel: [_ w1385 _] -> w1279
          tunnel: [_ _ w1413] -> w1276
          tunnel: [_ w1366 _] -> w1277
          tunnel: [_ w1397 _] -> w1278
          tunnel: w1282 -> [w1299 _ _]
          tunnel: w1281 -> [_ _ w1414]
          tunnel: [w1290 _ _] -> w1280
          frame #0 {
            n738 = local read "fab1_totalWt"() -> (w1293:sgl)
            n739 = local read "fab3_totalWt"() -> (w1295:sgl)
            n740 = local read "fab5_totalWt"() -> (w1297:sgl)
            n741 = local read "fab2_totalWt"() -> (w1294:sgl)
            n742 = local read "fab4_totalWt"() -> (w1296:sgl)
            n743 = local read "fab6_totalWt"() -> (w1298:sgl)
            n744 = Build Array(w1293, w1294, w1295, w1296, w1297, w1298) -> (w1292:sgl[])
            n745 = for {
              tunnel: w1299 -> [w1302] mode=indexing
              tunnel: w1292 -> [w1303] mode=indexing
              tunnel: [w1304] -> w1291 mode=indexing
              # "FABRIC"
              n746 = Unbundle By Name(w1302) -> ("Number of Plies"=w1301:i32)
              n747 = Less Or Equal To 0?(x=w1301) -> (x <= 0?=w1300:bool)
              n748 = case shown="False" w1300 {
                tunnel: [w1314 w1344] -> w1304
                tunnel: w1303 -> [w1311 _]
                tunnel: w1302 -> [w1305 _]
                frame False {
                  n749 = Unbundle By Name(w1305) -> ("Number of Plies"=w1316:i32, "Fabric.vendor"=w1330:u16, "Fabric.styleNum"=w1329:u16, "Fabric.fiber"=w1328:u16, "Fabric.denier"=w1327:u16, "Fabric.pickWeave"=w1326:u16, "Fabric.finish"=w1325:u16, "LotNum"=w1318:string, "RollNum"=w1317:string, "ozPerYd2"=w1313:sgl, "Fabric.stitch"=w1308:u16)
                  n750 = To Long Integer(number=w1308) -> (32bit integer=w1310:i32)
                  n751 = To Long Integer(number=w1330) -> (32bit integer=w1342:i32)
                  n752 = To Long Integer(number=w1329) -> (32bit integer=w1337:i32)
                  n753 = To Long Integer(number=w1328) -> (32bit integer=w1338:i32)
                  n754 = To Long Integer(number=w1327) -> (32bit integer=w1336:i32)
                  n755 = To Long Integer(number=w1326) -> (32bit integer=w1335:i32)
                  n756 = To Long Integer(number=w1325) -> (32bit integer=w1331:i32)
                  n757 = property on="Fabric.stitch" class="Ring (strict)"() -> ("Strings []"=w1309:string[])  [unwired: 2 in, 2 out]
                  n758 = Format Into String(w1316) -> (resulting string=w1315:string)  [unwired: 3 in, 1 out]
                  n759 = property on="Fabric.styleNum" class="Ring (strict)"() -> ("Strings []"=w1339:string[])  [unwired: 2 in, 2 out]
                  n760 = property on="Fabric.denier" class="Ring (strict)"() -> ("Strings []"=w1334:string[])  [unwired: 2 in, 2 out]
                  n761 = property on="Fabric.vendor" class="Ring (strict)"() -> ("Strings []"=w1341:string[])  [unwired: 2 in, 2 out]
                  n762 = property on="Fabric.fiber" class="Ring (strict)"() -> ("Strings []"=w1340:string[])  [unwired: 2 in, 2 out]
                  n763 = property on="Fabric.pickWeave" class="Ring (strict)"() -> ("Strings []"=w1333:string[])  [unwired: 2 in, 2 out]
                  n764 = property on="Fabric.finish" class="Ring (strict)"() -> ("Strings []"=w1332:string[])  [unwired: 2 in, 2 out]
                  n765 = Format Into String(w1313) -> (resulting string=w1312:string)  [unwired: 3 in, 1 out]
                  n766 = Format Into String(w1311) -> (resulting string=w1307:string)  [unwired: 3 in, 1 out]
                  n767 = Index Array(array=w1309, index=w1310) -> (element=w1306:string)
                  n768 = Index Array(array=w1341, index=w1342) -> (element=w1324:string)
                  n769 = Index Array(array=w1339, index=w1337) -> (element=w1323:string)
                  n770 = Index Array(array=w1340, index=w1338) -> (element=w1322:string)
                  n771 = Index Array(array=w1334, index=w1336) -> (element=w1321:string)
                  n772 = Index Array(array=w1333, index=w1335) -> (element=w1320:string)
                  n773 = Index Array(array=w1332, index=w1331) -> (element=w1319:string)
                  n774 = Build Array(w1315, w1324, w1323, w1322, w1321, w1320, w1319, w1318, w1317, w1312, w1307, w1306) -> (w1314:string[])
                }
                frame True {
                  n775 = call <vilib>:"Space Constant.vi"() -> ("String"=w1345:string)
                  n776 = Initialize Array(w1345, 12 ("dimension size")) -> (w1344:string[])
                }
              }
            }
            n777 = Transpose 2D Array(2D array=w1291) -> (transposed array=w1290:string[][])
          }
          frame #1 {
            w1398 = "%1d" ("format string")
            # "THREAT"
            # "SAMPLE"
            # "RANGE"
            # "RESULTS"
            n778 = local read "rangeOfResults"() -> (w1403:i32)
            n779 = local read "computed_V50"() -> (w1406:sgl)
            n780 = local read "lowComplete"() -> (w1404:i32)
            n781 = local read "highPartial"() -> (w1405:i32)
            n782 = local read "totalSampleWt"() -> (w1374:sgl)
            n783 = control-ref of="Panel Dimensions"() -> (w1382:refnum<vi>)
            n784 = control-ref of="workType"() -> (w1383:refnum<vi>)
            n785 = control-ref of="covering"() -> (w1384:refnum<vi>)
            n786 = local read "modelNum"() -> (w1376:string)
            n787 = local read "Sample ID"() -> (w1380:string)
            n788 = local read "serialNum"() -> (w1377:string)
            n789 = local read "zmr 2"() -> (w1402:sgl)
            n790 = local read "Thickness"() -> (w1371:dbl)
            n791 = local read "totalBAW"() -> (w1370:sgl)
            n792 = local read "minV50"() -> (w1367:i32)
            n793 = call "Dropdown Selection (SubVI).vi"("reference"=w1382) -> ("element"=w1379:string)
            n794 = call "Dropdown Selection (SubVI).vi"("reference"=w1383) -> ("element"=w1378:string)
            n795 = call "Dropdown Selection (SubVI).vi"("reference"=w1384) -> ("element"=w1375:string)
            n796 = Format Into String(format string="%1.1f", w1406) -> (resulting string=w1411:string)  [unwired: 2 in, 1 out]
            n797 = Format Into String(format string=w1398, w1405) -> (resulting string=w1410:string)  [unwired: 2 in, 1 out]
            n798 = Format Into String(format string=w1398, w1404) -> (resulting string=w1409:string)  [unwired: 2 in, 1 out]
            n799 = Format Into String(format string=w1398, w1403) -> (resulting string=w1412:string)  [unwired: 2 in, 1 out]
            n800 = Format Into String(format string="%1.1f", w1402) -> (resulting string=w1408:string)  [unwired: 2 in, 1 out]
            n801 = Format Into String(w1374) -> (resulting string=w1373:string)  [unwired: 3 in, 1 out]
            n802 = Format Into String(w1371) -> (resulting string=w1372:string)  [unwired: 3 in, 1 out]
            n803 = Format Into String(w1370) -> (resulting string=w1369:string)  [unwired: 3 in, 1 out]
            n804 = Format Into String(w1367) -> (resulting string=w1368:string)  [unwired: 3 in, 1 out]
            n805 = Bundle(w1411, w1410, w1409, w1412, w1408) -> (w1407:cluster{string, string, string, string, string})  [unwired: 1 in]
            n806 = Bundle("Sample ID"=w1380, "element"=w1379, "element"=w1378, "serialNum"=w1377, "modelNum"=w1376, w1373, w1372, w1369, "element"=w1375, w1368) -> (w1381:T13)  [unwired: 1 in]
            n807 = Cluster To Array(cluster=w1407) -> (array=w1401:string[])
            n808 = Cluster To Array(cluster=w1381) -> (array=w1366:string[])
            n809 = Build Array(w1401) -> (w1397:string[][])
            n810 = local read "Room Temperature"() -> (w1390:i32)
            n811 = local read "Room Humidity"() -> (w1389:i32)
            n812 = local read "clayAverage"() -> (w1394:sgl)
            n813 = local read "Shot Angle"() -> (w1347:u16)
            n814 = local read "clayTemp"() -> (w1392:i16)
            n815 = local read "clayCalib"() -> (w1395:string)
            n816 = control-ref of="weapon"() -> (w1362:refnum<vi>)
            n817 = control-ref of="projectile"() -> (w1361:refnum<vi>)
            n818 = control-ref of="weight(gr)"() -> (w1358:refnum<vi>)
            n819 = control-ref of="Powder Type"() -> (w1359:refnum<vi>)
            n820 = control-ref of="barrelLen"() -> (w1360:refnum<vi>)
            n821 = control-ref of="rangeNum"() -> (w1363:refnum<vi>)
            n822 = control-ref of="shooter"() -> (w1365:refnum<vi>)
            n823 = control-ref of="recorder"() -> (w1364:refnum<vi>)
            n824 = Format Into String(w1389) -> (resulting string=w1387:string)  [unwired: 3 in, 1 out]
            n825 = Format Into String(w1390) -> (resulting string=w1388:string)  [unwired: 3 in, 1 out]
            n826 = Format Into String(format string="%d", w1392) -> (resulting string=w1391:string)  [unwired: 2 in, 1 out]
            n827 = Format Into String(w1394) -> (resulting string=w1393:string)  [unwired: 3 in, 1 out]
            n828 = Format Into String(w1347) -> (resulting string=w1348:string)  [unwired: 3 in, 1 out]
            n829 = call "Dropdown Selection (SubVI).vi"("reference"=w1362) -> ("element"=w1356:string)
            n830 = call "Dropdown Selection (SubVI).vi"("reference"=w1361) -> ("element"=w1355:string)
            n831 = call "Dropdown Selection (SubVI).vi"("reference"=w1358) -> ("element"=w1354:string)
            n832 = call "Dropdown Selection (SubVI).vi"("reference"=w1359) -> ("element"=w1353:string)
            n833 = call "Dropdown Selection (SubVI).vi"("reference"=w1360) -> ("element"=w1352:string)
            n834 = call "Dropdown Selection (SubVI).vi"("reference"=w1363) -> ("element"=w1351:string)
            n835 = call "Dropdown Selection (SubVI).vi"("reference"=w1365) -> ("element"=w1350:string)
            n836 = call "Dropdown Selection (SubVI).vi"("reference"=w1364) -> ("element"=w1349:string)
            n837 = Bundle(w1387, w1388, w1391, "clayCalib"=w1395, w1393) -> (w1396:T14)  [unwired: 1 in]
            n838 = Bundle("element"=w1356, "element"=w1355, "element"=w1354, "element"=w1353, "element"=w1352, w1348, "element"=w1351, "element"=w1350, "element"=w1349) -> (w1357:T15)  [unwired: 1 in]
            n839 = Cluster To Array(cluster=w1396) -> (array=w1385:string[])
            n840 = Cluster To Array(cluster=w1357) -> (array=w1346:string[])
          }
          frame #2 {
            # "SHOT TABLE"
            n841 = for {
              tunnel: w1414 -> [w1436] mode=indexing
              tunnel: [w1415] -> w1413 mode=indexing
              n842 = Unbundle By Name(w1436) -> ("shot order"=w1435:i32, "Powder Loading"=w1434:sgl, "Uncorrected Impact"=w1433:sgl, "UncorrectedRed_PB"=w1432:sgl, "UncorrectedAvgVel_PB"=w1431:sgl, "velLoss_PB"=w1430:sgl, "strikeVel_PB"=w1429:sgl, "SHOT STATUS"=w1417:u16, "usedv50"=w1427:bool, "BackFace\nDepth"=w1428:sgl)
              n843 = case shown="1" w1417 {
                tunnel: ["P" "C"] -> w1416
                frame 0, Default {
                }
                frame 1 {
                }
              }
              n844 = case shown="True" w1427 {
                tunnel: ["" ("Empty String Constant") "*"] -> w1426
                frame False {
                }
                frame True {
                }
              }
              n845 = Format Into String(w1435) -> (resulting string=w1419:string)  [unwired: 3 in, 1 out]
              n846 = Format Into String(w1434) -> (resulting string=w1420:string)  [unwired: 3 in, 1 out]
              n847 = Format Into String(w1433) -> (resulting string=w1421:string)  [unwired: 3 in, 1 out]
              n848 = Format Into String(w1432) -> (resulting string=w1422:string)  [unwired: 3 in, 1 out]
              n849 = Format Into String(w1431) -> (resulting string=w1423:string)  [unwired: 3 in, 1 out]
              n850 = Format Into String(w1430) -> (resulting string=w1424:string)  [unwired: 3 in, 1 out]
              n851 = Format Into String(w1429) -> (resulting string=w1425:string)  [unwired: 3 in, 1 out]
              n852 = Format Into String(w1428) -> (resulting string=w1418:string)  [unwired: 3 in, 1 out]
              n853 = Build Array(w1419, w1420, w1421, w1422, w1423, w1424, w1425, w1416, w1426, w1418) -> (w1415:string[])
            }
          }
        }
        n854 = local read "Test Comments"() -> (w1271:string)
        n855 = control-ref of="Method"() -> (w1286:refnum<vi>)
        n856 = control-ref of="standard"() -> (w1285:refnum<vi>)
        n857 = local read "projName"() -> (w1273:string)
        n858 = local read "projNum"() -> (w1272:string)
        n859 = call "Dropdown Selection (SubVI).vi"("reference"=w1286) -> ("element"=w1274:string)
        n860 = call "Dropdown Selection (SubVI).vi"("reference"=w1285) -> ("element"=w1270:string)
        n861 = To Variant(anything=w1280) -> (Variant=w1269:variant)
        n862 = To Variant(anything=w1279) -> (Variant=w1268:variant)
        n863 = To Variant(anything=w1278) -> (Variant=w1267:variant)
        n864 = To Variant(anything=w1277) -> (Variant=w1266:variant)
        n865 = To Variant(anything=w1276) -> (Variant=w1265:variant)
        n866 = To Variant(anything=w1275) -> (Variant=w1264:variant)
        n867 = To Variant(anything=w1274) -> (Variant=w1263:variant)
        n868 = To Variant(anything=w1273) -> (Variant=w1262:variant)
        n869 = To Variant(anything=w1272) -> (Variant=w1261:variant)
        n870 = To Variant(anything=w1271) -> (Variant=w1260:variant)
        n871 = To Variant(anything=w1270) -> (Variant=w1259:variant)
        n872 = call "MS Office Report2"("Enable"=w1284, "blockFabric"=w1269, "blockRange"=w1268, "blockResults"=w1267, "blockSample"=w1266, "blockShotTbl"=w1265, "blockThreat"=w1264, "method"=w1263, "projName"=w1262, "projNum"=w1261, "remark"=w1260, "standard"=w1259) -> ("error out"=w1283:errorcluster)  [unwired: 15 in]
        n873 = call <vilib>:"Simple Error Handler.vi"("error in (no error)"=w1283) -> ("error out"=w1287:errorcluster)  [unwired: 4 in, 4 out]
        n874 = case shown="No Error" w1287 {
          frame No Error {
            n875 = One Button Dialog(message="A Ballistic Test  Report is ready.") -> ()  [unwired: 1 in, 1 out]
          }
          frame Error {
          }
        }
      }
    }
  }
